vi "Start_10_July.vi"() -> ()   [LabVIEW 2015]
uses:
  gfitsio/gfitsio-refnum.ctl
  SystemUtil/Command.ctl
  Instance          11 21Saved   Start_10_July .vi
  Instance          12 21Saved   Start_10_July .vi
panel:
  in  "Zoom Window Width (1/x)":u32=10
  out "max index(es)":i32
  out "max index(es) 2":i32
  in  "Resolution Factor":u16=4
  out "Spectrum Status":string
  out "Image Buffer Info.":T1
  out "error IO":errorcluster
  out "Raw Spectrum Array":dbl[](array[numeric])
  in  "# of rows at a time":dbl=1.0
  in  "Black Square":picture
  in  "Image Buffer":i32[][](array[numeric])
  out "Column Cut Cursor Position":dbl
  out "Raw Image Buffer 1":i16[][](array[numeric])
  out "Raw Data":T2
  out "gfits refnum":T3
  in  "Tab Control":T4(tab)
  in  "Autoscale":bool
  in  "Image Display Resolution":u16(ring)=2 items=["High", "Medium", "Low"]
  in  "Send Object Offset Position":bool
  in  "Send Target Offset Position":bool
  in  "Automatic Acquisition?":bool=TRUE caption="Display:"
  in  "Display Directions?":bool caption="Display:"
  in  "Redraw":bool
  in  "Zoom Out":bool
  in  "Zoom In":bool
  out "Y":dbl format="%5.1f"
  out "X":dbl format="%5.1f"
  out "Value":dbl
  out "Zoom Window":i16[][](graph) caption="0051.NGC2808_300line.fits"
  out "Compass":picture
  out "Image Status":string
  in  "Image Scale Stretch":cluster{dbl, dbl}(slide)={0.0, 1.4018691588785046} scale=0.0..100.0
  in  "Image":dbl[][](graph)=[[10.0, 5.0, 0.0], [0.0, 6.0, 7.0]] caption="Image Buffer"
  out "Calib Spec":cluster{dbl, dbl}[](graph) caption="Spectrum Centered at Row 53"
  in  "Show x scale in:":i32(listbox)
  in  "Refresh Spectrum":bool
  in  "Aperture Width (pix)":dbl=5.0
  out "Cut Along Column":i16[](graph)
  in  "Cut Along Column #":dbl min=0.0 max=2071.0
  in  "Refresh Spatial Cut":bool
  out "Minimum Pix Value":dbl
  out "Maximum Pix Value":dbl
  out "Avg Pix Value":dbl format="%#.1f"
  in  "Header Scroll":dbl(slide)=100.0 scale=0.0..100.0
  out "FITS Header":string[](array[string])
  in  "CommandQ":string="QUICKLOOK_Q"
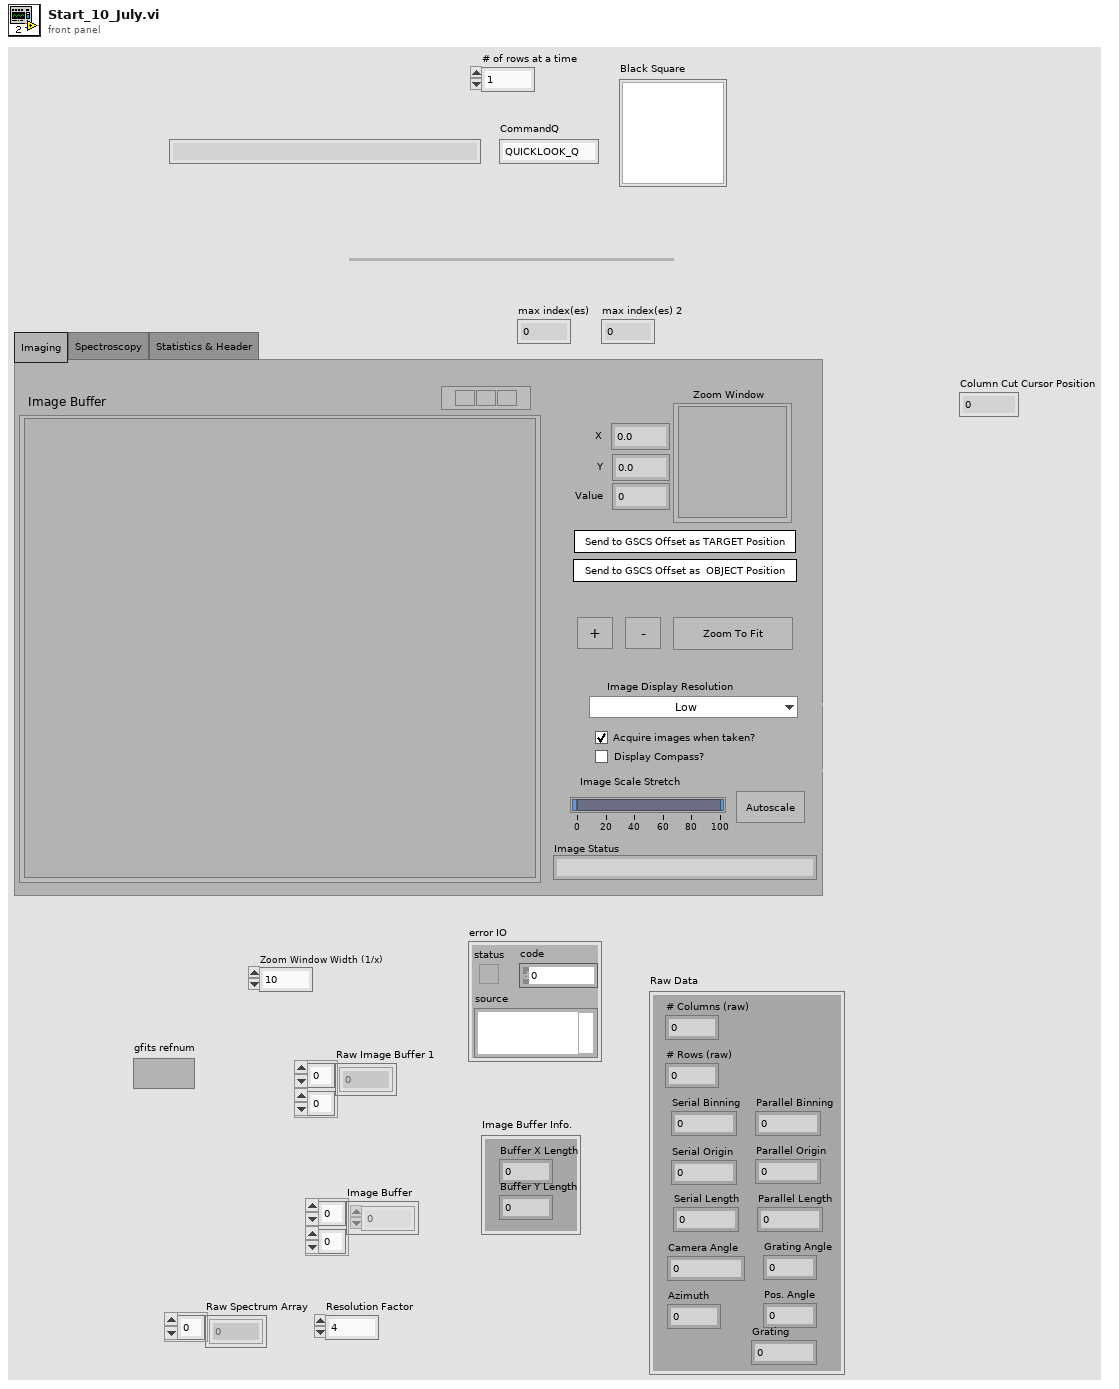
[diagram p1: front panel]
types:
  T1 = cluster{"Buffer X Length":dbl, "Buffer Y Length ":dbl}
  T2 = cluster{"# Columns (raw) ":dbl, "# Rows (raw)":dbl, "Serial Origin":dbl, "Parallel Origin":dbl, "Camera Angle":dbl, "Grating Angle":dbl, "Serial Binning":dbl, "Parallel Binning":dbl, "Azimuth":dbl, "Serial Length":dbl, "Parallel Length":dbl, "Pos. Angle":dbl, "Grating":dbl}
  T3 = typedef "gfitsio-refnum.ctl" = refnum<k1>
  T4 = enum32{"Imaging", "Spectroscopy", "Statistics & Header"}
  T5 = typedef "Command.ctl" = cluster{"Command":string, "Parameter":string}
  T6 = enum16{"open", "open or create", "create or replace", "create", "open (read only)"}
  T7 = cluster{"Width":u16, "Style":enum32{"Solid", "Dash", "Dot", "DashDot", "DashDotDot"}}
  T8 = enum32{"existing file", "new file", "new or existing file", "existing dir", "new dir", "new or existing dir", "existing file (use LLBs)", "new file (use LLBs)", "new or existing file (use LLBs)", "new or existing file or directory (use LLBs)"}
  T9 = typedef "LVRangeTypeDef.ctl" = cluster{"Minimum":dbl, "Maximum":dbl, "Increment":dbl, "Minor Increment":dbl, "Start":dbl}
  T10 = typedef "LVPoint32TypeDef.ctl" = cluster{"Horizontal":i32, "Vertical":i32}
  T11 = typedef "LVPointDoubleTypeDef.ctl" = cluster{"Cursor X":dbl, "Cursor Y":dbl}
  T12 = cluster{"Font Name:":string, "Size":i16, "Strikeout?":bool, "Italic?":bool, "Underline?":bool, "Outline?":bool, "Shadow?":bool, "Bold?":bool}
  T13 = cluster{"horizontal":enum16{"left", "center", "right"}, "vertical":enum16{"top", "center", "bottom"}}
  T14 = enum16{"User-specified Font", "Application Font", "System Font", "Dialog Font"}
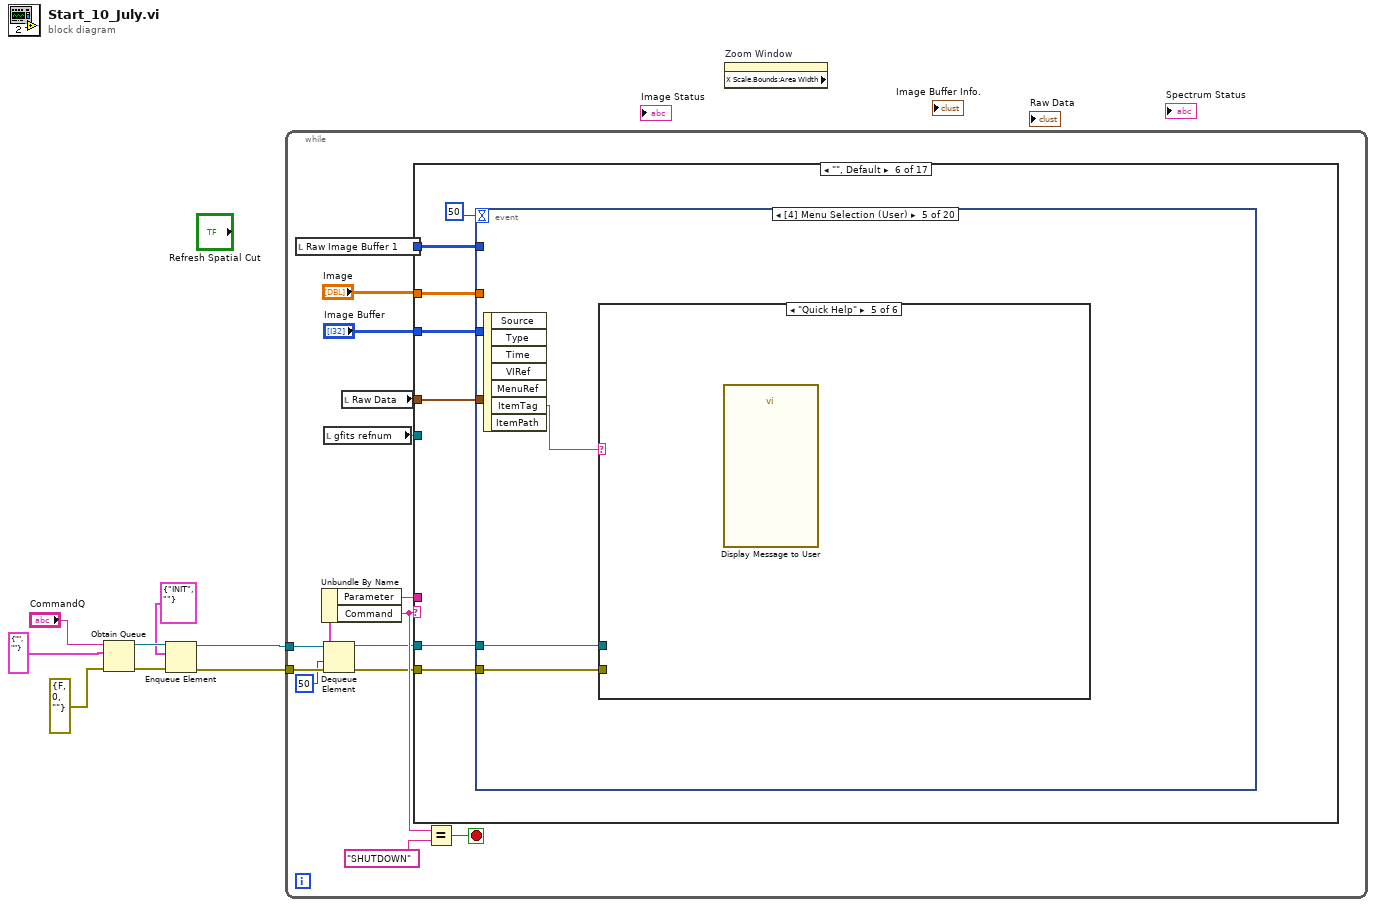
[diagram p0: block diagram]
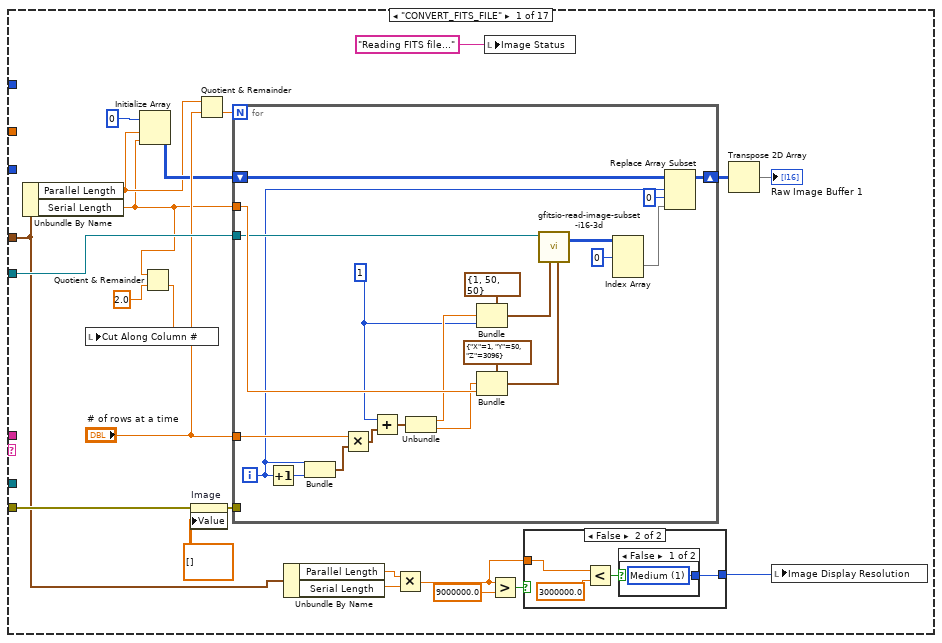
[diagram p2: hidden frame]
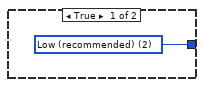
[diagram p3: hidden frame]
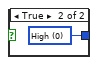
[diagram p4: hidden frame]
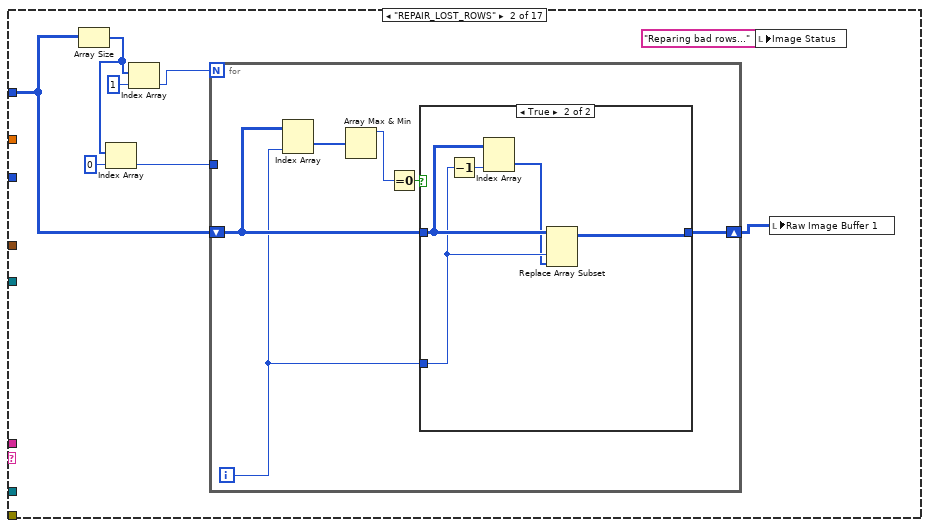
[diagram p5: hidden frame]
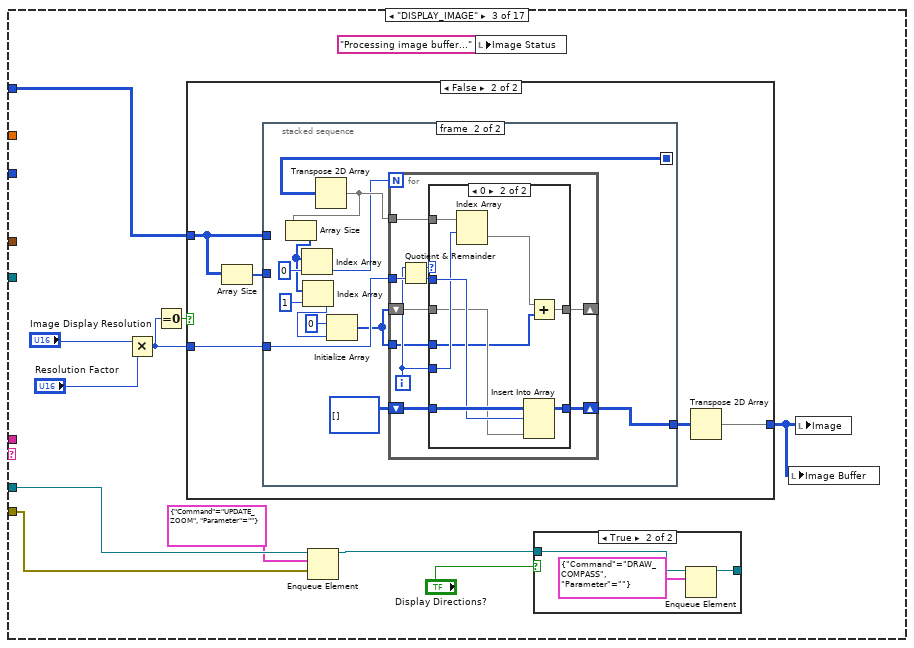
[diagram p7: hidden frame]
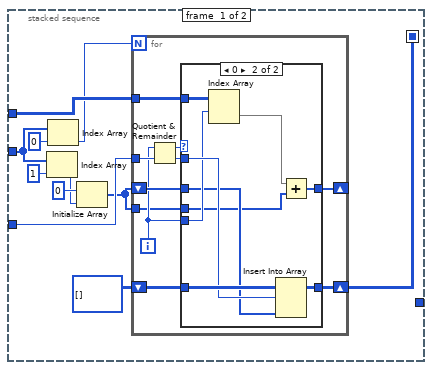
[diagram p10: hidden frame]
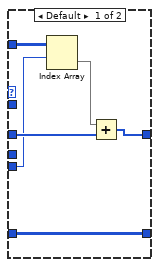
[diagram p11: hidden frame]
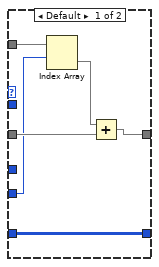
[diagram p12: hidden frame]
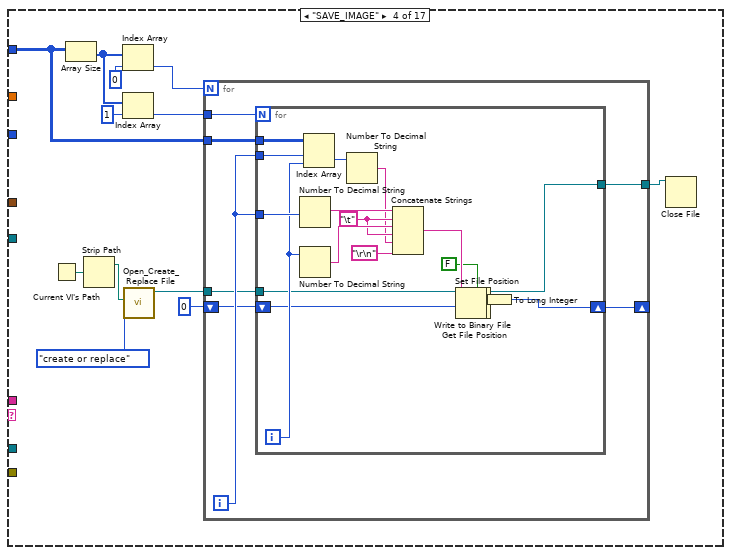
[diagram p13: hidden frame]
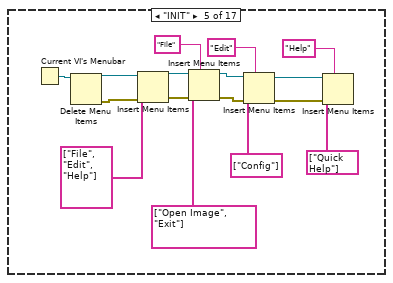
[diagram p14: hidden frame]
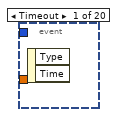
[diagram p15: hidden frame]
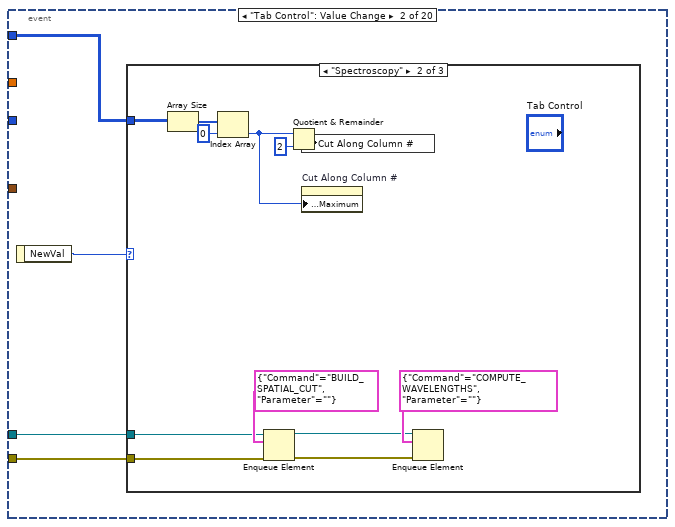
[diagram p16: hidden frame]
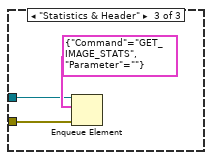
[diagram p18: hidden frame]
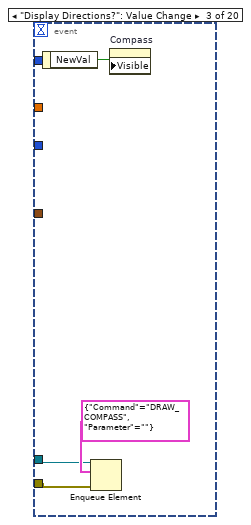
[diagram p19: hidden frame]
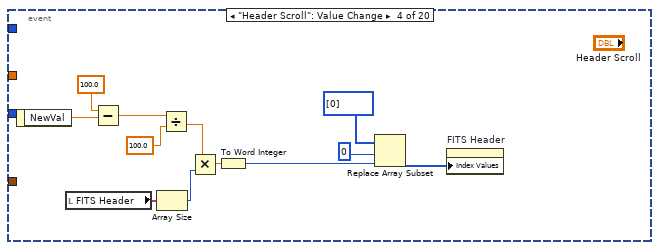
[diagram p20: hidden frame]
diagram:
  n1 = Obtain Queue(name (unnamed)="CommandQ", element data type=T5 {"Command"="", "Parameter"=""} ("Command"), error in (no error)=errorcluster {"status"=FALSE, "code"=0, "source"=""}) -> (queue out=w6:refnum<queue>, error out=w5:errorcluster)  [unwired: 2 in, 1 out]
  n2 = Enqueue Element(queue=w6, element=T5 {"Command"="INIT", "Parameter"=""}, error in (no error)=w5) -> (queue out=w3:refnum<queue>, error out=w2:errorcluster)  [unwired: 1 in, 1 out]
  n3 = while {
    tunnel: w2 -> [w23]
    tunnel: w3 -> [w22]
    stop <- w19 stop-if-true
    n4 = local read "Raw Image Buffer 1"() -> (w9:i16[][])
    n5 = local read "gfits refnum"() -> (w13:T3)
    n6 = Dequeue Element(queue=w22, timeout in ms (-1)=50, error in (no error)=w23) -> (queue out=w16:refnum<queue>, element=w21:T5, error out=w17:errorcluster)  [unwired: 1 out]
    n7 = Unbundle By Name(w21) -> ("Parameter"=w14:string, "Command"=w18:string)
    n8 = local read "Raw Data"() -> (w12:T2)
    n9 = case shown="\"\", Default" w18 {
      tunnel: w17 -> [w36 _ w94 _ _ w249 w652 _ _ _ _ _ _ _ w990 w1020 _]
      tunnel: w16 -> [_ _ w97 _ _ w250 w653 _ _ _ _ _ _ _ w989 _ _]
      tunnel: w14 -> [_ _ _ _ _ _ _ _ _ _ _ _ _ _ w988 _ _]
      tunnel: "Image" -> [_ _ _ _ _ w248 _ _ _ _ _ _ _ _ _ _ _]
      tunnel: w13 -> [w45 _ _ _ _ _ _ _ _ _ _ _ _ _ _ w1021 _]
      tunnel: w12 -> [w30 _ _ _ _ w247 w651 _ _ _ w841 w909 _ w971 _ w1018 _]
      tunnel: "Image Buffer" -> [_ _ _ _ _ w246 _ _ _ _ _ _ _ _ _ _ _]
      tunnel: w9 -> [_ w78 w101 w198 _ w245 _ _ w777 w783 _ _ w964 w967 _ _ w1091]
      frame "CONVERT_FITS_FILE" {
        n10 = Unbundle By Name(w30) -> ("Parallel Length"=w32:dbl, "Serial Length"=w31:dbl)
        n11 = Initialize Array(i16 0 ("element"), w32, w31) -> (w34:i16[][])
        n12 = Quotient & Remainder(x=w31, y=2.0) -> (floor(x/y)=w39:dbl)  [unwired: 1 out]
        n13 = local write "Cut Along Column #"(w39) -> ()
        n14 = property on="Image" class="IntGraph (strict)"(error in=w36, "Value"=dbl[][] [] ("Image")) -> (error out=w37:errorcluster)  [unwired: 1 in, 1 out]
        n15 = Quotient & Remainder(x=w32, y="# of rows at a time") -> (floor(x/y)=w44:dbl)  [unwired: 1 out]
        n16 = for {
          N: w44 -> [_]
          tunnel: w31 -> [w72]
          tunnel: w45 -> [w61]
          tunnel: "# of rows at a time" -> [w71]
          shift-right: [w57] -> w41
          shift-left: w34 -> [w56]
          tunnel: w37 -> [_]
          i -> [w55]
          w64 = 1
          n17 = Increment(x=w55) -> (x+1=w68:i32)
          n18 = Bundle(w55, w68) -> (w69:cluster{i32, i32})  [unwired: 1 in]
          n19 = Multiply(x=w71, y=w69) -> (x*y=w70:cluster{dbl, dbl})
          n20 = Add(x=w64, y=w70) -> (x+y=w67:cluster{dbl, dbl})
          n21 = Unbundle(w67) -> (w65:dbl, w66:dbl)
          n22 = Bundle(cluster=cluster{"X":i32, "Y":i32, "Z":i32} {"X"=1, "Y"=50, "Z"=50} ("fpixel (1,1,1)"), "Y"=w65, "Z"=w64) -> (w60:cluster{"X":i32, "Y":i32, "Z":i32})  [unwired: 1 in]
          n23 = Bundle(cluster=cluster{"X":i32, "Y":i32, "Z":i32} {"X"=1, "Y"=50, "Z"=3096} ("lpixel (-1,-1,-1: rest)"), "Y"=w66, "Z"=w72) -> (w59:cluster{"X":i32, "Y":i32, "Z":i32})  [unwired: 1 in]
          n24 = call "gfitsio-read-image-subset-i16-3d.vi"("lpixel (-1,-1,-1: rest)"=w59, "fpixel (1,1,1)"=w60, "gfits refnum"=w61) -> ("data"=w58:i16[][][])  [unwired: 5 in, 3 out]
          n25 = Index Array(array=w58, index (dim 0)=i16 0 ("index (page)")) -> (element=w54:i16[][])  [unwired: 2 in]
          n26 = Replace Array Subset(array=w56, new element=w54, index (row)=w55, index (col)=0 ("disabled index (col)")) -> (w57:i16[][])
        }
        n27 = Unbundle By Name(w30) -> ("Parallel Length"=w29:dbl, "Serial Length"=w28:dbl)
        n28 = Multiply(x=w29, y=w28) -> (x*y=w24:dbl)
        n29 = local write "Image Status"("Reading FITS file..." ("Status")) -> ()
        n30 = Greater?(x=w24, y=9000000.0) -> (0:w26:bool)
        n31 = case shown="False" w26 {
          tunnel: [w46 w47] -> w25
          tunnel: w24 -> [_ w49]
          frame True {
            w46 = u16 2 items=["High", "Medium", "Low (recommended)"] ("Image Display Resolution")
          }
          frame False {
            n32 = Less?(x=w49, y=3000000.0) -> (x < y?=w50:bool)
            n33 = case shown="False" w50 {
              tunnel: [w51 w52] -> w47
              frame False {
                w51 = u16 1 items=["High", "Medium", "Low (recommended)"] ("Image Display Resolution")
              }
              frame True {
                w52 = u16 0 items=["High", "Medium", "Low (recommended)"] ("Image Display Resolution")
              }
            }
          }
        }
        n34 = Transpose 2D Array(2D array=w41) -> (transposed array=→"Raw Image Buffer 1":i16[][])
        n35 = local write "Image Display Resolution"(w25) -> ()
      }
      frame "REPAIR_LOST_ROWS" {
        n36 = Array Size(array=w78) -> (size(s)=w75:i32[])
        n37 = Index Array(array=w75, index=0) -> (element=w74:i32)
        n38 = Index Array(array=w75, index=1) -> (element=w79:i32)
        n39 = for {
          N: w79 -> [_]
          shift-right: [w87] -> w80
          shift-left: w78 -> [w86]
          tunnel: w74 -> [_]
          i -> [w85]
          n40 = Index Array(array=w86, index (col)=w85) -> (element=w84:i16[])  [unwired: 1 in]
          n41 = Array Max & Min(array=w84) -> (max value=w82:i16)  [unwired: 3 out]
          n42 = Equal To 0?(x=w82) -> (x = 0?=w83:bool)
          n43 = case shown="True" w83 {
            tunnel: w85 -> [_ w90]
            tunnel: w86 -> [w88 w92]
            tunnel: [w88 w93] -> w87
            frame False {
            }
            frame True {
              n44 = Decrement(x=w90) -> (x-1=w91:i32)
              n45 = Index Array(array=w92, index (col)=w91) -> (element=w89:i16[])  [unwired: 1 in]
              n46 = Replace Array Subset(array=w92, new element=w89, index (col)=w90) -> (w93:i16[][])  [unwired: 1 in]
            }
          }
        }
        n47 = local write "Image Status"("Reparing bad rows..." ("Image Status")) -> ()
        n48 = local write "Raw Image Buffer 1"(w80) -> ()
      }
      frame "DISPLAY_IMAGE" {
        n49 = Multiply(x="Image Display Resolution", y="Resolution Factor") -> (x*y=w102:u16)
        n50 = Equal To 0?(x=w102) -> (x = 0?=w103:bool)
        n51 = case shown="False" w103 {
          tunnel: w101 -> [w110 w114]
          tunnel: w102 -> [_ w112]
          tunnel: [w110 w111] -> w99
          frame True {
          }
          frame False {
            n52 = Array Size(array=w114) -> (size(s)=w115:i32[])
            n53 = stacked-sequence {
              seq-local: [w124 _] -> [_ w161]
              tunnel: w114 -> [w126 _]
              tunnel: w115 -> [w118 _]
              tunnel: w112 -> [w122 w158]
              tunnel: [_ w162] -> w113
              frame #0 {
                n54 = Index Array(array=w118, index=1) -> (element=w117:i32)
                n55 = Index Array(array=w118, index=0) -> (element=w120:i32)
                n56 = Initialize Array(0 ("element"), w117) -> (w116:i32[])
                n57 = for {
                  N: w120 -> [_]
                  tunnel: w126 -> [w136]
                  shift-right: [w134] -> w124
                  shift-left: i32[][] [] -> [w135]
                  tunnel: w122 -> [w133]
                  shift-right: [w129] -> _
                  shift-left: w116 -> [w130]
                  tunnel: w116 -> [w127]
                  i -> [w128]
                  n58 = Quotient & Remainder(x=w128, y=w133) -> (x-y*floor(x/y)=w132:i32, floor(x/y)=w131:i32)
                  n59 = case shown="0" w132 {
                    tunnel: w136 -> [w142 w151]
                    tunnel: w128 -> [w138 w147]
                    tunnel: w135 -> [w137 w150]
                    tunnel: [w137 w149] -> w134
                    tunnel: w131 -> [_ w148]
                    tunnel: w130 -> [w140 w146]
                    tunnel: [w139 w144] -> w129
                    tunnel: w127 -> [_ w143]
                    frame Default {
                      n60 = Index Array(array=w142, index (row)=w138) -> (element=w141:i16[])  [unwired: 1 in]
                      n61 = Add(x=w141, y=w140) -> (x+y=w139:i32[])
                    }
                    frame 0 {
                      n62 = Index Array(array=w151, index (row)=w147) -> (element=w145:i16[])  [unwired: 1 in]
                      n63 = Insert Into Array(array=w150, index (row)=w148, new element=w146) -> (w149:i32[][])  [unwired: 1 in]
                      n64 = Add(x=w145, y=w143) -> (x+y=w144:i32[])
                    }
                  }
                }
              }
              frame #1 {
                n65 = Transpose 2D Array(2D array=w161) -> (transposed array=w159:i32[][])
                n66 = Array Size(array=w159) -> (size(s)=w153:i32[])
                n67 = Index Array(array=w153, index=0) -> (element=w156:i32)
                n68 = Index Array(array=w153, index=1) -> (element=w154:i32)
                n69 = Initialize Array(0 ("element"), w154) -> (w152:i32[])
                n70 = for {
                  N: w156 -> [_]
                  tunnel: w159 -> [w173]
                  shift-right: [w166] -> w162
                  shift-left: i32[][] [] -> [w167]
                  shift-right: [w172] -> _
                  shift-left: w152 -> [w171]
                  tunnel: w158 -> [w168]
                  tunnel: w152 -> [w164]
                  i -> [w165]
                  n71 = Quotient & Remainder(x=w165, y=w168) -> (x-y*floor(x/y)=w170:i32, floor(x/y)=w169:i32)
                  n72 = case shown="0" w170 {
                    tunnel: w173 -> [w179 w188]
                    tunnel: w165 -> [w175 w184]
                    tunnel: w167 -> [w174 w187]
                    tunnel: [w174 w186] -> w166
                    tunnel: w169 -> [_ w185]
                    tunnel: w171 -> [w177 w183]
                    tunnel: [w176 w181] -> w172
                    tunnel: w164 -> [_ w180]
                    frame Default {
                      n73 = Index Array(array=w179, index (row)=w175) -> (element=w178:i32[])  [unwired: 1 in]
                      n74 = Add(x=w178, y=w177) -> (x+y=w176:i32[])
                    }
                    frame 0 {
                      n75 = Index Array(array=w188, index (row)=w184) -> (element=w182:i32[])  [unwired: 1 in]
                      n76 = Insert Into Array(array=w187, index (row)=w185, new element=w183) -> (w186:i32[][])  [unwired: 1 in]
                      n77 = Add(x=w182, y=w180) -> (x+y=w181:i32[])
                    }
                  }
                }
              }
            }
            n78 = Transpose 2D Array(2D array=w113) -> (transposed array=w111:i32[][])
          }
        }
        n79 = Enqueue Element(queue=w97, element=T5 {"Command"="UPDATE_ZOOM", "Parameter"=""}, error in (no error)=w94) -> (queue out=w96:refnum<queue>)  [unwired: 1 in, 2 out]
        n80 = local write "Image Status"("Processing image buffer..." ("Status")) -> ()
        n81 = case shown="True" "Display Directions?" {
          tunnel: w96 -> [w106 w108]
          tunnel: [w106 w107] -> _
          frame False {
          }
          frame True {
            n82 = Enqueue Element(queue=w108, element=T5 {"Command"="DRAW_COMPASS", "Parameter"=""}) -> (queue out=w107:refnum<queue>)  [unwired: 2 in, 2 out]
          }
        }
        n83 = local write "Image Buffer"(w99) -> ()
        n84 = local write "Image"(w99) -> ()
      }
      frame "SAVE_IMAGE" {
        n85 = Current VI's Path() -> (path=w193:path)
        n86 = Array Size(array=w198) -> (size(s)=w196:i32[])
        n87 = Strip Path(path=w193) -> (stripped path=w192:path)  [unwired: 1 out]
        n88 = Index Array(array=w196, index=0) -> (element=w199:i32)
        n89 = Index Array(array=w196, index=1) -> (element=w195:i32)
        n90 = call <vilib>:"Open_Create_Replace File.vi"("function (open:0)"=T6."create or replace", "start path  (Not A Path)"=w192) -> ("refnum"=w191:refnum<file>)  [unwired: 6 in, 3 out]
        n91 = for {
          N: w199 -> [_]
          tunnel: w198 -> [w207]
          tunnel: w195 -> [w206]
          tunnel: w191 -> [w204]
          tunnel: [w203] -> w190
          shift-right: [w201] -> _
          shift-left: 0 ("pos offset (0)") -> [w202]
          i -> [w205]
          n92 = for {
            N: w206 -> [_]
            tunnel: w207 -> [w228]
            tunnel: w205 -> [w227]
            tunnel: w205 -> [w226]
            tunnel: w204 -> [w218]
            tunnel: [w217] -> w203
            shift-right: [w215] -> w201
            shift-left: w202 -> [w216]
            i -> [w221]
            w223 = "\t"
            n93 = Number To Decimal String(number=w226) -> (decimal integer string=w225:string)  [unwired: 1 in]
            n94 = Number To Decimal String(number=w221) -> (decimal integer string=w224:string)  [unwired: 1 in]
            n95 = Index Array(array=w228, index (row)=w227, index (col)=w221) -> (element=w222:i16)
            n96 = Number To Decimal String(number=w222) -> (decimal integer string=w220:string)  [unwired: 1 in]
            n97 = Concatenate Strings(w225, w223, w224, w223, w220, "\r\n") -> (w219:string)
            n98 = Set File Position(offset (in bytes) (0)=w216, refnum=w218) -> (refnum out=w213:refnum<file>, error out=w212:errorcluster)  [unwired: 2 in]
            n99 = Write to Binary File(file (use dialog)=w213, data=w219, error in=w212, 5:FALSE ("prepend array or string size? (T)")) -> (refnum out=w211:refnum<file>, error out=w210:errorcluster)  [unwired: 2 in, 1 out]
            n100 = Get File Position(4:w210, 7:w211) -> (2:w209:i64, 3:w217:refnum<file>)  [unwired: 1 out]
            n101 = To Long Integer(number=w209) -> (32bit integer=w215:i32)
          }
        }
        n102 = Close File(refnum=w190) -> ()  [unwired: 1 in, 2 out]
      }
      frame "INIT" {
        n103 = Current VI's Menubar() -> (w244:refnum<k9>)
        n104 = Delete Menu Items(9:w244) -> (0:w242:errorcluster, 3:w243:refnum<k9>)  [unwired: 3 in]
        n105 = Insert Menu Items(6:w242, 8:string[] ["File", "Edit", "Help"] ("item names"), 9:w243) -> (0:w237:errorcluster, 3:w240:refnum<k9>)  [unwired: 3 in, 1 out]
        n106 = Insert Menu Items(5:"File" ("menu tag"), 6:w237, 8:string[] ["Open Image", "Exit"] ("item names"), 9:w240) -> (0:w235:errorcluster, 3:w236:refnum<k9>)  [unwired: 2 in, 1 out]
        n107 = Insert Menu Items(5:"Edit" ("menu tag"), 6:w235, 8:string[] ["Config"] ("item names"), 9:w236) -> (0:w231:errorcluster, 3:w232:refnum<k9>)  [unwired: 2 in, 1 out]
        n108 = Insert Menu Items(5:"Help" ("menu tag"), 6:w231, 8:string[] ["Quick Help"] ("item names"), 9:w232) -> ()  [unwired: 2 in, 3 out]
      }
      frame "", Default {
        n109 = event shown="[4] Menu Selection (User)" {
          selector: _ -> [_ _ _ _ _ _ _ _ _ _ _ _ _ _ _ _ _ _ _ _]
          dyn-events: _ -> [_ _ _ _ _ _ _ _ _ _ _ _ _ _ _ _ _ _ _ _]
          timeout: 50 -> [_ _ _ _ _ _ _ _ _ _ _ _ _ _ _ _ _ _ _ _]
          tunnel: w250 -> [_ w253 w271 _ w288 _ w317 w320 w324 _ _ _ _ w587 w596 w613 w615 w618 _ w648]
          tunnel: w249 -> [_ w254 w272 _ w287 _ w318 w321 w325 _ _ _ _ w588 w598 w612 w616 w619 _ w647]
          tunnel: w248 -> [_ _ _ _ _ _ _ _ w326 _ _ _ _ _ _ _ _ w620 _ _]
          tunnel: w247 -> [_ _ _ _ _ _ _ _ w323 _ _ _ _ _ _ _ _ _ _ _]
          tunnel: w246 -> [_ _ _ _ _ _ _ _ _ _ _ _ _ _ _ _ _ _ _ _]
          tunnel: w245 -> [_ w252 _ _ _ _ _ _ _ _ _ _ _ _ _ _ _ _ _ _]
          event Timeout {
            n110 = event-data() -> ()  [unwired: 1 in, 2 out]
          }
          event "Tab Control": Value Change {
            n111 = event-data() -> ("NewVal"=w255:T4)  [unwired: 1 in]
            n112 = case shown="\"Spectroscopy\"" w255 {
              tunnel: w252 -> [_ w267 _]
              tunnel: w254 -> [_ w260 w269]
              tunnel: w253 -> [_ w259 w268]
              frame "Imaging", Default {
              }
              frame "Spectroscopy" {
                n113 = Array Size(array=w267) -> (size(s)=w266:i32[])
                n114 = Index Array(array=w266, index=0) -> (element=w262:i32)
                n115 = Enqueue Element(queue=w259, element=T5 {"Command"="BUILD_SPATIAL_CUT", "Parameter"=""}, error in (no error)=w260) -> (queue out=w256:refnum<queue>, error out=w257:errorcluster)  [unwired: 1 in, 1 out]
                n116 = Quotient & Remainder(x=w262, y=2) -> (floor(x/y)=w263:i32)  [unwired: 1 out]
                n117 = local write "Cut Along Column #"(w263) -> ()
                n118 = property on="Cut Along Column #" class="DigNum (strict)"("Data Entry Limits:Maximum"=w262) -> ()  [unwired: 2 in, 2 out]
                n119 = Enqueue Element(queue=w256, element=T5 {"Command"="COMPUTE_WAVELENGTHS", "Parameter"=""}, error in (no error)=w257) -> ()  [unwired: 1 in, 3 out]
              }
              frame "Statistics & Header" {
                n120 = Enqueue Element(queue=w268, element=T5 {"Command"="GET_IMAGE_STATS", "Parameter"=""}, error in (no error)=w269) -> ()  [unwired: 1 in, 3 out]
              }
            }
          }
          event "Display Directions?": Value Change {
            n121 = event-data() -> ("NewVal"=w274:bool)  [unwired: 1 in]
            n122 = Enqueue Element(queue=w271, element=T5 {"Command"="DRAW_COMPASS", "Parameter"=""}, error in (no error)=w272) -> ()  [unwired: 1 in, 3 out]
            n123 = property on="Compass" class="Pict"("Visible"=w274) -> ()  [unwired: 2 in, 2 out]
          }
          event "Header Scroll": Value Change {
            n124 = event-data() -> ("NewVal"=w284:dbl)  [unwired: 1 in]
            n125 = local read "FITS Header"() -> (w286:string[])
            n126 = Subtract(x=100.0, y=w284) -> (x-y=w276:dbl)
            n127 = Array Size(array=w286) -> (size(s)=w283:i32)
            n128 = Divide(x=w276, y=100.0) -> (x/y=w275:dbl)
            n129 = Multiply(x=w275, y=w283) -> (x*y=w279:dbl)
            n130 = To Word Integer(number=w279) -> (16bit integer=w278:i16)
            n131 = Replace Array Subset(array=u32[] [0] ("Index Values"), new element=w278, index=0) -> (w280:u32[])
            n132 = property on="FITS Header" class="Arr (strict)"("Index Values"=w280) -> ()  [unwired: 2 in, 2 out]
          }
          event Menu Selection (User) {
            n133 = event-data() -> ("ItemTag"=w289:string)  [unwired: 1 in, 6 out]
            n134 = case shown="\"Quick Help\"" w289 {
              tunnel: w288 -> [_ w292 w300 _ _ w313]
              tunnel: w287 -> [_ w291 w301 _ _ w312]
              frame "", Default {
              }
              frame "Exit" {
                n135 = Enqueue Element(queue=w292, element=T5 {"Command"="SHUTDOWN", "Parameter"=""}, error in (no error)=w291) -> ()  [unwired: 1 in, 3 out]
              }
              frame "Open Image" {
                (unwired) T8."existing file" ("select mode (2)")
                n136 = File Dialog(5:"Open Image" ("button label"), 6:"*.fits" ("default name"), 7:"Open Image" ("prompt")) -> (0:w293:errorcluster, 1:w297:bool, 3:w298:path)  [unwired: 4 in, 1 out]
                n137 = Unbundle(w293) -> ()  [unwired: 3 out]
                n138 = Path To String(path=w298) -> (string=w299:string)
                n139 = case shown="False" w297 {
                  tunnel: w301 -> [_ w307]
                  tunnel: w300 -> [_ w306]
                  tunnel: w299 -> [_ w304]
                  frame True {
                  }
                  frame False {
                    n140 = Bundle By Name(cluster=T5 {"Command"="", "Parameter"=""} ("element"), "Command"="OPEN_FITS_FILE", "Parameter"=w304) -> (w305:T5)
                    n141 = Enqueue Element(queue=w306, element=w305, error in (no error)=w307) -> ()  [unwired: 1 in, 3 out]
                  }
                }
              }
              frame "Config" {
                n142 = call "Configuration Parameters"() -> ("Rows to read in at a time"=w310:dbl)  [unwired: 15 in, 4 out]
                n143 = Equal To 0?(x=w310) -> (x = 0?=w311:bool)
                n144 = Select(t=5.0, s=w311, f=w310) -> (s? t:f=w308:dbl)
                n145 = local write "# of rows at a time"(w308) -> ()
              }
              frame "Quick Help" {
                n146 = call "Display Message to User"() -> ()  [unwired: 10 in, 2 out]
              }
              frame "Save" {
                n147 = Enqueue Element(queue=w313, element=T5 {"Command"="SAVE_IMAGE", "Parameter"=""}, error in (no error)=w312) -> ()  [unwired: 1 in, 3 out]
              }
            }
          }
          event "Autoscale": Value Change {
            n148 = event-data() -> ()  [unwired: 1 in, 6 out]
            n149 = property on="Image" class="IntGraph (strict)"("Z Scale.Scale Fit"=u8 1) -> ()  [unwired: 2 in, 2 out]
            n150 = local write "Autoscale"(FALSE ("Autoscale")) -> ()
          }
          event "Image Display Resolution": Value Change {
            n151 = event-data() -> ()  [unwired: 1 in, 6 out]
            n152 = Enqueue Element(queue=w317, element=T5 {"Command"="DISPLAY_IMAGE", "Parameter"=""}, error in (no error)=w318) -> ()  [unwired: 1 in, 3 out]
          }
          event "Redraw": Mouse Down {
            n153 = event-data() -> ()  [unwired: 1 in, 8 out]
            n154 = Enqueue Element(queue=w320, element=T5 {"Command"="DISPLAY_IMAGE", "Parameter"=""}, error in (no error)=w321) -> ()  [unwired: 1 in, 3 out]
          }
          event Key Down {
            n155 = event-data() -> ("Char"=w327:i16)  [unwired: 1 in]
            n156 = case shown="116" w327 {
              selector: w327 -> [_ _ w342 _ _ _ _ _]
              tunnel: w326 -> [_ _ _ _ _ _ _ _]
              tunnel: w325 -> [_ _ w338 w361 w430 _ w490 _]
              tunnel: w324 -> [_ _ w337 w362 w431 _ w489 _]
              tunnel: w323 -> [_ _ _ _ _ _ _ _]
              frame 0 {
              }
              frame Default {
              }
              frame 105..108 {
                w332 = u16 1 ("t")
                n157 = local read "Image Display Resolution"() -> (w335:u16)
                n158 = local read "Resolution Factor"() -> (w328:u16)
                n159 = property on="Image" class="IntGraph (strict)"() -> ("Cursor.Cursor Position:Cursor X"=w330:dbl)  [unwired: 2 in, 2 out]
                n160 = property on="Image" class="IntGraph (strict)"() -> ("Cursor.Cursor Position:Cursor Y"=w329:dbl)  [unwired: 2 in, 2 out]
                n161 = Enqueue Element(queue=w337, element=T5 {"Command"="UPDATE_ZOOM", "Parameter"=""}, error in (no error)=w338) -> ()  [unwired: 1 in, 3 out]
                n162 = Multiply(x=w335, y=w328) -> (x*y=w336:u16)
                n163 = Equal To 0?(x=w335) -> (x = 0?=w334:bool)
                n164 = Select(t=w332, s=w334, f=w336) -> (s? t:f=w333:u16)
                n165 = Divide(x=w332, y=w333) -> (x/y=w331:dbl)
                n166 = case shown="105" w342 {
                  tunnel: w330 -> [w344 w347 w352 w355 w360]
                  tunnel: [w344 w346 w352 w354 w360] -> w341
                  tunnel: w329 -> [w343 w348 w350 w356 w358]
                  tunnel: [w343 w348 w349 w356 w357] -> w340
                  tunnel: w331 -> [_ w345 w351 w353 w359]
                  frame 0, Default {
                  }
                  frame 108 {
                    n167 = Add(x=w347, y=w345) -> (x+y=w346:dbl)
                  }
                  frame 105 {
                    n168 = Add(x=w350, y=w351) -> (x+y=w349:dbl)
                  }
                  frame 106 {
                    n169 = Subtract(x=w355, y=w353) -> (x-y=w354:dbl)
                  }
                  frame 107 {
                    n170 = Subtract(x=w358, y=w359) -> (x-y=w357:dbl)
                  }
                }
                n171 = property on="Image" class="IntGraph (strict)"("Cursor.Cursor Position:Cursor X"=w341) -> ()  [unwired: 2 in, 2 out]
                n172 = property on="Image" class="IntGraph (strict)"("Cursor.Cursor Position:Cursor Y"=w340) -> ()  [unwired: 2 in, 2 out]
              }
              frame 114 {
                n173 = local read "Zoom Window"() -> (w368:i16[][])
                n174 = Array Size(array=w368) -> (size(s)=w364:i32[])
                n175 = Index Array(array=w364, index=1) -> (element=w363:i32)
                n176 = Index Array(array=w364, index=0) -> (element=w366:i32)
                n177 = stacked-sequence {
                  seq-local: [w369 _ _ _] -> [_ _ w407 _]
                  seq-local: [_ w382 _ _] -> [_ _ w408 _]
                  seq-local: [_ _ w395 _] -> [_ _ _ w422]
                  tunnel: w368 -> [w375 w386 _ _]
                  tunnel: w366 -> [w372 w385 _ _]
                  tunnel: w363 -> [w371 w384 _ _]
                  tunnel: w362 -> [_ _ _ w418]
                  tunnel: w361 -> [_ _ _ w417]
                  frame #0 {
                    n178 = Initialize Array(0 ("element"), w371) -> (w374:i32[])
                    n179 = for {
                      N: w372 -> [_]
                      tunnel: w375 -> [w381]
                      shift-right: [w380] -> w370
                      shift-left: w374 -> [w378]
                      i -> [w376]
                      n180 = Index Array(array=w381, index (row)=w376) -> (element=w379:i16[])  [unwired: 1 in]
                      n181 = Add(x=w379, y=w378) -> (x+y=w377:i32[])
                      n182 = Replace Array Subset(array=w378, new element=w377) -> (w380:i32[])  [unwired: 1 in]
                    }
                    n183 = Array Max & Min(array=w370) -> (max index (indices)=w369:i32)  [unwired: 3 out]
                  }
                  frame #1 {
                    n184 = Initialize Array(0 ("element"), w385) -> (w388:i32[])
                    n185 = for {
                      N: w384 -> [_]
                      tunnel: w386 -> [w394]
                      shift-right: [w393] -> w383
                      shift-left: w388 -> [w390]
                      i -> [w389]
                      n186 = Index Array(array=w394, index (col)=w389) -> (element=w391:i16[])  [unwired: 1 in]
                      n187 = Add(x=w391, y=w390) -> (x+y=w392:i32[])
                      n188 = Replace Array Subset(array=w390, new element=w392) -> (w393:i32[])  [unwired: 1 in]
                    }
                    n189 = Array Max & Min(array=w383) -> (max index (indices)=w382:i32)  [unwired: 3 out]
                  }
                  frame #2 {
                    n190 = property on="Zoom Window" class="IntGraph (strict)"() -> ("Y Scale.Range:Minimum"=w400:dbl)  [unwired: 2 in, 2 out]
                    n191 = property on="Zoom Window" class="IntGraph (strict)"() -> ("X Scale.Range:Maximum"=w402:dbl)  [unwired: 2 in, 2 out]
                    n192 = property on="Zoom Window" class="IntGraph (strict)"() -> ("X Scale.Range:Minimum"=w403:dbl)  [unwired: 2 in, 2 out]
                    n193 = property on="Zoom Window" class="IntGraph (strict)"() -> ("Y Scale.Range:Maximum"=w401:dbl)  [unwired: 2 in, 2 out]
                    n194 = Subtract(x=w401, y=w400) -> (x-y=w406:dbl)
                    n195 = Subtract(x=w402, y=w403) -> (x-y=w405:dbl)
                    n196 = Bundle(w405, w406) -> (w409:cluster{dbl, dbl})  [unwired: 1 in]
                    n197 = local read "X"() -> (w413:dbl)
                    n198 = local read "Y"() -> (w412:dbl)
                    n199 = Divide(x=w409, y=2) -> (x/y=w404:cluster{dbl, dbl})
                    n200 = Bundle(w408, w407) -> (w411:cluster{i32, i32})  [unwired: 1 in]
                    n201 = Bundle("X"=w413, "Y"=w412) -> (w410:cluster{"X":dbl, "Y":dbl})  [unwired: 1 in]
                    n202 = Subtract(x=w411, y=w404) -> (x-y=w398:cluster{dbl, dbl})
                    n203 = To Word Integer(number=w398) -> (16bit integer=w399:cluster{i16, i16})
                    n204 = To Double Precision Float(number=w399) -> (double precision float=w397:cluster{dbl, dbl})
                    n205 = Add(x=w397, y=w410) -> (x+y=w396:cluster{dbl, dbl})
                    n206 = To Word Integer(number=w396) -> (16bit integer=w395:cluster{i16, i16})
                  }
                  frame #3 {
                    n207 = local read "Image Display Resolution"() -> (w426:u16)
                    n208 = Enqueue Element(queue=w418, element=T5 {"Command"="ZOOM_FOR_GAUSS_FIT", "Parameter"=""}, error in (no error)=w417) -> (queue out=w415:refnum<queue>, error out=w416:errorcluster)  [unwired: 1 in, 1 out]
                    n209 = local read "Resolution Factor"() -> (w429:u16)
                    n210 = Enqueue Element(queue=w415, element=T5 {"Command"="FIT_GAUSSIAN", "Parameter"=""}, error in (no error)=w416) -> ()  [unwired: 1 in, 3 out]
                    n211 = Multiply(x=w426, y=w429) -> (x*y=w427:u16)
                    n212 = Equal To 0?(x=w426) -> (x = 0?=w424:bool)
                    n213 = Select(t=u16 1, s=w424, f=w427) -> (s? t:f=w428:u16)
                    n214 = To Double Precision Float(number=w428) -> (double precision float=w423:dbl)
                    n215 = Divide(x=w422, y=w423) -> (x/y=w421:cluster{dbl, dbl})
                    n216 = property on="Image" class="IntGraph (strict)"("Cursor.Cursor Position"=w421) -> ()  [unwired: 2 in, 2 out]
                  }
                }
              }
              frame 97 {
                n217 = local read "Zoom Window"() -> (w432:i16[][])
                n218 = Array Size(array=w432) -> (size(s)=w436:i32[])
                n219 = Index Array(array=w436, index=1) -> (element=w437:i32)
                n220 = Index Array(array=w436, index=0) -> (element=w434:i32)
                n221 = stacked-sequence {
                  seq-local: [w440 _ _] -> [_ w453 _]
                  seq-local: [_ w456 _] -> [_ _ w464]
                  tunnel: w432 -> [w444 _ _]
                  tunnel: w434 -> [w438 _ _]
                  tunnel: w437 -> [w439 _ _]
                  tunnel: w431 -> [_ _ w461]
                  tunnel: w430 -> [_ _ w462]
                  frame #0 {
                    n222 = Initialize Array(0 ("element"), w438) -> (w443:i32[])
                    n223 = for {
                      N: w439 -> [_]
                      tunnel: w444 -> [w450]
                      shift-right: [w449] -> w441
                      shift-left: w443 -> [w447]
                      i -> [w445]
                      n224 = Index Array(array=w450, index (col)=w445) -> (element=w448:i16[])  [unwired: 1 in]
                      n225 = Add(x=w448, y=w447) -> (x+y=w446:i32[])
                      n226 = Replace Array Subset(array=w447, new element=w446) -> (w449:i32[])  [unwired: 1 in]
                    }
                    n227 = Array Max & Min(array=w441) -> (max index (indices)=w440:i32)  [unwired: 3 out]
                  }
                  frame #1 {
                    n228 = property on="Zoom Window" class="IntGraph (strict)"() -> ("X Scale.Range:Minimum"=w454:dbl)  [unwired: 2 in, 2 out]
                    n229 = property on="Zoom Window" class="IntGraph (strict)"() -> ("X Scale.Range:Maximum"=w455:dbl)  [unwired: 2 in, 2 out]
                    n230 = Subtract(x=w455, y=w454) -> (x-y=w452:dbl)
                    n231 = Divide(x=w452, y=2) -> (x/y=w458:dbl)
                    n232 = local read "X"() -> (w451:dbl)
                    n233 = Subtract(x=w453, y=w458) -> (x-y=w457:dbl)
                    n234 = Add(x=w457, y=w451) -> (x+y=w456:dbl)
                  }
                  frame #2 {
                    n235 = local read "Image Display Resolution"() -> (w468:u16)
                    n236 = local read "Resolution Factor"() -> (w471:u16)
                    n237 = Enqueue Element(queue=w461, element=T5 {"Command"="UPDATE_ZOOM", "Parameter"=""}, error in (no error)=w462) -> ()  [unwired: 1 in, 3 out]
                    n238 = Multiply(x=w468, y=w471) -> (x*y=w469:u16)
                    n239 = Equal To 0?(x=w468) -> (x = 0?=w466:bool)
                    n240 = Select(t=u16 1, s=w466, f=w469) -> (s? t:f=w470:u16)
                    n241 = To Double Precision Float(number=w470) -> (double precision float=w465:dbl)
                    n242 = Divide(x=w464, y=w465) -> (x/y=w460:dbl)
                    n243 = property on="Image" class="IntGraph (strict)"("Cursor.Cursor Position:Cursor X"=w460) -> ()  [unwired: 2 in, 2 out]
                  }
                }
              }
              frame 116 {
                n244 = local write "Tab Control"(T4."Imaging" ("Tab Control")) -> ()
              }
              frame 115 {
                n245 = local read "Image Display Resolution"() -> (w482:u16)
                n246 = property on="Image" class="IntGraph (strict)"() -> ("Cursor.Cursor Position:Cursor Y"=w477:dbl)  [unwired: 2 in, 2 out]
                n247 = Enqueue Element(queue=w489, element=T5 {"Command"="BUILD_SPATIAL_CUT", "Parameter"=""}, error in (no error)=w490) -> (queue out=w486:refnum<queue>, error out=w487:errorcluster)  [unwired: 1 in, 1 out]
                n248 = Multiply(x=w482, y=u16 4) -> (x*y=w483:u16)
                n249 = Equal To 0?(x=w482) -> (x = 0?=w480:bool)
                n250 = Select(t=u16 1, s=w480, f=w483) -> (s? t:f=w484:u16)
                n251 = To Double Precision Float(number=w484) -> (double precision float=w478:dbl)
                n252 = local write "Tab Control"(T4."Spectroscopy" ("Tab Control")) -> ()
                n253 = Multiply(x=w477, y=w478) -> (x*y=w476:dbl)
                n254 = Enqueue Element(queue=w486, element=T5 {"Command"="BUILD_SPECTRUM", "Parameter"=""}, error in (no error)=w487) -> (queue out=w473:refnum<queue>, error out=w474:errorcluster)  [unwired: 1 in, 1 out]
                n255 = local write "Column Cut Cursor Position"(w476) -> ()
                n256 = Enqueue Element(queue=w473, element=T5 {"Command"="COMPUTE_WAVELENGTHS", "Parameter"=""}, error in (no error)=w474) -> ()  [unwired: 1 in, 3 out]
              }
              frame 99 {
                n257 = property on="Image" class="IntGraph (strict)"() -> ("X Scale.Range:Maximum"=w498:dbl)  [unwired: 2 in, 2 out]
                n258 = property on="Image" class="IntGraph (strict)"() -> ("Y Scale.Range:Maximum"=w500:dbl)  [unwired: 2 in, 2 out]
                n259 = property on="Image" class="IntGraph (strict)"() -> ("Y Scale.Range:Minimum"=w499:dbl)  [unwired: 2 in, 2 out]
                n260 = property on="Image" class="IntGraph (strict)"() -> ("X Scale.Range:Minimum"=w497:dbl)  [unwired: 2 in, 2 out]
                n261 = Subtract(x=w498, y=w497) -> (x-y=w496:dbl)
                n262 = Subtract(x=w500, y=w499) -> (x-y=w495:dbl)
                n263 = Bundle(w496, w495) -> (w494:cluster{dbl, dbl})  [unwired: 1 in]
                n264 = Divide(x=w494, y=2) -> (x/y=w492:cluster{dbl, dbl})
                n265 = property on="Image" class="IntGraph (strict)"("Cursor.Cursor Position"=w492) -> ()  [unwired: 2 in, 2 out]
              }
            }
          }
          event "Send Target Offset Position": Value Change {
            w507 = " " ("string")
            n266 = event-data() -> ()  [unwired: 1 in, 1 out]
            n267 = local read "X"() -> (w515:dbl)
            n268 = local read "Y"() -> (w514:dbl)
            n269 = Format Into String(w515) -> (resulting string=w513:string)  [unwired: 3 in, 1 out]
            n270 = Format Into String(w514) -> (resulting string=w512:string)  [unwired: 3 in, 1 out]
            n271 = Concatenate Strings("T" ("string"), w507, w513, w507, w512) -> (w510:string)
            n272 = Bundle("Command"="ACCEPT_OFFSET_COORD", w510) -> (w502:cluster{"Command":string, string})  [unwired: 1 in]
            n273 = Obtain Queue(name (unnamed)="SICAMERA_Command_Q", element data type=T5 {"Command"="", "Parameter"=""} ("element")) -> (queue out=w505:refnum<queue>, created new?=w504:bool, error out=w503:errorcluster)  [unwired: 3 in]
            n274 = case shown="False" w504 {
              tunnel: w502 -> [_ w523]
              tunnel: w505 -> [_ w522]
              tunnel: w503 -> [_ w521]
              tunnel: ["Error upon sending the offset coord." ("Image Status") "Coordinates successfully uploaded to GSCS!" ("Image Status")] -> w501
              frame True {
              }
              frame False {
                n275 = Enqueue Element(queue=w522, element=w523, error in (no error)=w521) -> (queue out=w520:refnum<queue>, error out=w519:errorcluster)  [unwired: 1 in, 1 out]
                n276 = Release Queue(queue=w520, error in (no error)=w519) -> ()  [unwired: 1 in, 3 out]
              }
            }
            n277 = local write "Send Target Offset Position"(FALSE ("Send Target Offset Position")) -> ()
            n278 = local write "Image Status"(w501) -> ()
          }
          event "Send Object Offset Position": Value Change {
            w527 = " " ("string")
            n279 = event-data() -> ()  [unwired: 1 in, 1 out]
            n280 = local read "X"() -> (w539:dbl)
            n281 = local read "Y"() -> (w538:dbl)
            n282 = Format Into String(w539) -> (resulting string=w537:string)  [unwired: 3 in, 1 out]
            n283 = Format Into String(w538) -> (resulting string=w536:string)  [unwired: 3 in, 1 out]
            n284 = Concatenate Strings("O" ("string"), w527, w537, w527, w536) -> (w534:string)
            n285 = Obtain Queue(name (unnamed)="SICAMERA_Command_Q", element data type=T5 {"Command"="", "Parameter"=""} ("element")) -> (queue out=w532:refnum<queue>, created new?=w525:bool, error out=w531:errorcluster)  [unwired: 3 in]
            n286 = Bundle("Command"="ACCEPT_OFFSET_COORD", w534) -> (w533:cluster{"Command":string, string})  [unwired: 1 in]
            n287 = case shown="True" w525 {
              tunnel: w533 -> [_ w546]
              tunnel: w532 -> [_ w545]
              tunnel: w531 -> [_ w544]
              tunnel: ["Error upon sending the offset coord." ("Image Status") "Coordinates successfully uploaded to GSCS!" ("Image Status")] -> w524
              frame True {
              }
              frame False {
                n288 = Enqueue Element(queue=w545, element=w546, error in (no error)=w544) -> (queue out=w543:refnum<queue>, error out=w542:errorcluster)  [unwired: 1 in, 1 out]
                n289 = Release Queue(queue=w543, error in (no error)=w542) -> ()  [unwired: 1 in, 3 out]
              }
            }
            n290 = local write "Send Object Offset Position"(FALSE ("Send Object Offset Position")) -> ()
            n291 = local write "Image Status"(w524) -> ()
          }
          event "Zoom In": Mouse Down {
            n292 = event-data() -> ()  [unwired: 1 in, 8 out]
            n293 = property on="Image" class="IntGraph (strict)"() -> ("X Scale.Range"=w566:T9)  [unwired: 2 in, 2 out]
            n294 = property on="Image" class="IntGraph (strict)"() -> ("Y Scale.Range"=w565:T9)  [unwired: 2 in, 2 out]
            n295 = Unbundle By Name(w566) -> ("Maximum"=w564:dbl, "Minimum"=w558:dbl)
            n296 = Unbundle By Name(w565) -> ("Maximum"=w557:dbl, "Minimum"=w547:dbl)
            n297 = Subtract(x=w564, y=w558) -> (x-y=w563:dbl)
            n298 = Subtract(x=w557, y=w547) -> (x-y=w562:dbl)
            n299 = Bundle(w563, w562) -> (w559:cluster{dbl, dbl})  [unwired: 1 in]
            n300 = Bundle("Minimum"=w558, "Minimum"=w547) -> (w555:cluster{"Minimum":dbl, "Minimum":dbl})  [unwired: 1 in]
            n301 = Multiply(x=w559, y=0.5) -> (x*y=w553:cluster{dbl, dbl})
            n302 = Multiply(x=w559, y=0.25) -> (x*y=w556:cluster{dbl, dbl})
            n303 = Add(x=w556, y=w555) -> (x+y=w554:cluster{dbl, dbl})
            n304 = Add(x=w553, y=w554) -> (x+y=w550:cluster{dbl, dbl})
            n305 = Unbundle(w554) -> (w552:dbl, w551:dbl)
            n306 = Unbundle(w550) -> (w549:dbl, w548:dbl)
            n307 = property on="Image" class="IntGraph (strict)"("Y Scale.Range:Minimum"=w551) -> ()  [unwired: 2 in, 2 out]
            n308 = property on="Image" class="IntGraph (strict)"("X Scale.Range:Minimum"=w552) -> ()  [unwired: 2 in, 2 out]
            n309 = property on="Image" class="IntGraph (strict)"("X Scale.Range:Maximum"=w549) -> ()  [unwired: 2 in, 2 out]
            n310 = property on="Image" class="IntGraph (strict)"("Y Scale.Range:Maximum"=w548) -> ()  [unwired: 2 in, 2 out]
          }
          event "Zoom Out": Mouse Down {
            n311 = event-data() -> ()  [unwired: 1 in, 8 out]
            n312 = property on="Image" class="IntGraph (strict)"() -> ("X Scale.Range"=w586:T9)  [unwired: 2 in, 2 out]
            n313 = property on="Image" class="IntGraph (strict)"() -> ("Y Scale.Range"=w585:T9)  [unwired: 2 in, 2 out]
            n314 = Unbundle By Name(w586) -> ("Maximum"=w584:dbl, "Minimum"=w578:dbl)
            n315 = Unbundle By Name(w585) -> ("Maximum"=w577:dbl, "Minimum"=w570:dbl)
            n316 = Subtract(x=w584, y=w578) -> (x-y=w583:dbl)
            n317 = Subtract(x=w577, y=w570) -> (x-y=w582:dbl)
            n318 = Bundle(w583, w582) -> (w579:cluster{dbl, dbl})  [unwired: 1 in]
            n319 = Bundle("Minimum"=w578, "Minimum"=w570) -> (w568:cluster{"Minimum":dbl, "Minimum":dbl})  [unwired: 1 in]
            n320 = Multiply(x=w579, y=2) -> (x*y=w569:cluster{dbl, dbl})
            n321 = Multiply(x=w569, y=0.25) -> (x*y=w567:cluster{dbl, dbl})
            n322 = Subtract(x=w568, y=w567) -> (x-y=w576:cluster{dbl, dbl})
            n323 = Add(x=w569, y=w576) -> (x+y=w573:cluster{dbl, dbl})
            n324 = Unbundle(w576) -> (w575:dbl, w574:dbl)
            n325 = Unbundle(w573) -> (w572:dbl, w571:dbl)
            n326 = property on="Image" class="IntGraph (strict)"("Y Scale.Range:Minimum"=w574) -> ()  [unwired: 2 in, 2 out]
            n327 = property on="Image" class="IntGraph (strict)"("X Scale.Range:Minimum"=w575) -> ()  [unwired: 2 in, 2 out]
            n328 = property on="Image" class="IntGraph (strict)"("X Scale.Range:Maximum"=w572) -> ()  [unwired: 2 in, 2 out]
            n329 = property on="Image" class="IntGraph (strict)"("Y Scale.Range:Maximum"=w571) -> ()  [unwired: 2 in, 2 out]
          }
          event "Refresh Spatial Cut": Value Change {
            n330 = event-data() -> ()  [unwired: 1 in, 6 out]
            n331 = Enqueue Element(queue=w587, element=T5 {"Command"="BUILD_SPATIAL_CUT", "Parameter"=""}, error in (no error)=w588) -> ()  [unwired: 1 in, 3 out]
          }
          event "Cut Along Column": Mouse Up {
            # "Remove rest of code (left) if not allowing clicking to create spectrum"
            n332 = event-data() -> ("Coords"=w608:T10)  [unwired: 1 in]
            n333 = Enqueue Element(queue=w596, element=T5 {"Command"="BUILD_SPECTRUM", "Parameter"=""}, error in (no error)=w598) -> (queue out=w595:refnum<queue>, error out=w597:errorcluster)  [unwired: 1 in, 1 out]
            n334 = Unbundle By Name(w608) -> ("Horizontal"=w607:i32)
            n335 = property on="Cut Along Column" class="WFGraph (strict)"() -> ("Plot Area:Size:Width"=w591:u32)  [unwired: 2 in, 2 out]
            n336 = property on="Cut Along Column" class="WFGraph (strict)"() -> ("X Scale.Position:Left"=w594:i32)  [unwired: 2 in, 2 out]
            n337 = Enqueue Element(queue=w595, element=T5 {"Command"="COMPUTE_WAVELENGTHS", "Parameter"=""}, error in (no error)=w597) -> ()  [unwired: 1 in, 3 out]
            n338 = Add(x=w594, y=9) -> (x+y=w592:i32)
            n339 = property on="Cut Along Column" class="WFGraph (strict)"() -> ("X Scale.Range:Maximum"=w604:dbl)  [unwired: 2 in, 2 out]
            n340 = property on="Cut Along Column" class="WFGraph (strict)"() -> ("X Scale.Range:Minimum"=w601:dbl)  [unwired: 2 in, 2 out]
            n341 = Subtract(x=w607, y=w592) -> (x-y=w606:i32)
            n342 = Subtract(x=w604, y=w601) -> (x-y=w603:dbl)
            n343 = Divide(x=w606, y=w591) -> (x/y=w605:dbl)
            n344 = property on="Cut Along Column" class="WFGraph (strict)"() -> ("Cursor.Cursor Position:Cursor X"=→"Column Cut Cursor Position":dbl)  [unwired: 2 in, 2 out]
            n345 = Multiply(x=w605, y=w603) -> (x*y=w602:dbl)
            n346 = Add(x=w602, y=w601) -> ()  [unwired: 1 out]
          }
          event "Refresh Spectrum": Value Change {
            n347 = event-data() -> ()  [unwired: 1 in, 6 out]
            n348 = Enqueue Element(queue=w613, element=T5 {"Command"="BUILD_SPECTRUM", "Parameter"=""}, error in (no error)=w612) -> (queue out=w609:refnum<queue>, error out=w610:errorcluster)  [unwired: 1 in, 1 out]
            n349 = Enqueue Element(queue=w609, element=T5 {"Command"="COMPUTE_WAVELENGTHS", "Parameter"=""}, error in (no error)=w610) -> ()  [unwired: 1 in, 3 out]
          }
          event "Show x scale in:": Value Change {
            n350 = event-data() -> ()  [unwired: 1 in, 1 out]
            n351 = Enqueue Element(queue=w615, element=T5 {"Command"="COMPUTE_WAVELENGTHS", "Parameter"=""}, error in (no error)=w616) -> ()  [unwired: 1 in, 3 out]
          }
          event "Image": Mouse Down {
            n352 = event-data() -> ("Coords"=w621:T10)  [unwired: 1 in, 3 out]
            n353 = stacked-sequence {
              tunnel: w621 -> [w642 _]
              tunnel: w620 -> [_ _]
              tunnel: w619 -> [_ w644]
              tunnel: w618 -> [_ w643]
              frame #0 {
                # "Useless code.  Get rid of if keeping reading of coordinates  by cursor."
                n354 = Unbundle By Name(w642) -> ("Horizontal"=w641:i32, "Vertical"=w633:i32)
                n355 = property on="Image" class="IntGraph (strict)"() -> ("X Scale.Position:Left"=w626:i32)  [unwired: 2 in, 2 out]
                n356 = property on="Image" class="IntGraph (strict)"() -> ("Y Scale.Position:Top"=w624:i32)  [unwired: 2 in, 2 out]
                n357 = property on="Image" class="IntGraph (strict)"() -> ("Y Scale.Bounds:Area Height"=w625:u32)  [unwired: 2 in, 2 out]
                n358 = property on="Image" class="IntGraph (strict)"() -> ("Y Scale.Range:Maximum"=w628:dbl)  [unwired: 2 in, 2 out]
                n359 = property on="Image" class="IntGraph (strict)"() -> ("Y Scale.Range:Minimum"=w629:dbl)  [unwired: 2 in, 2 out]
                n360 = property on="Image" class="IntGraph (strict)"() -> ("X Scale.Bounds:Area Width"=w632:u32)  [unwired: 2 in, 2 out]
                n361 = property on="Image" class="IntGraph (strict)"() -> ("X Scale.Range:Minimum"=w630:dbl)  [unwired: 2 in, 2 out]
                n362 = property on="Image" class="IntGraph (strict)"() -> ("X Scale.Range:Maximum"=w631:dbl)  [unwired: 2 in, 2 out]
                n363 = Subtract(x=w641, y=w626) -> (x-y=w640:i32)
                n364 = Subtract(x=w633, y=w624) -> (x-y=w634:i32)
                n365 = Divide(x=w640, y=w632) -> (x/y=w638:dbl)
                n366 = Divide(x=w634, y=w625) -> (x/y=w635:dbl)
                n367 = Subtract(x=w631, y=w630) -> (x-y=w639:dbl)
                n368 = Subtract(x=w628, y=w629) -> (x-y=w636:dbl)
                n369 = Multiply(x=w638, y=w639) -> (x*y=w637:dbl)
                n370 = Multiply(x=w635, y=w636) -> (x*y=w627:dbl)
                n371 = Add(x=w637, y=w630) -> (x+y=w623:dbl)
                n372 = property on="Image" class="IntGraph (strict)"("Cursor.Cursor Position:Cursor X"=w623) -> ()  [unwired: 2 in, 2 out]
                n373 = Subtract(x=w628, y=w627) -> (x-y=w622:dbl)
                n374 = property on="Image" class="IntGraph (strict)"("Cursor.Cursor Position:Cursor Y"=w622) -> ()  [unwired: 2 in, 2 out]
              }
              frame #1 {
                n375 = Enqueue Element(queue=w643, element=T5 {"Command"="UPDATE_ZOOM", "Parameter"=""}, error in (no error)=w644) -> ()  [unwired: 1 in, 3 out]
              }
            }
          }
          event "Cut Along Column": Mouse Enter {
            n376 = event-data() -> ()  [unwired: 1 in, 4 out]
            n377 = local write "Spectrum Status"("Click to create aperture and corresponding spectrum" ("Spectrum Status")) -> ()
          }
          event "Image Scale Stretch": Mouse Up {
            n378 = event-data() -> ()  [unwired: 1 in, 9 out]
            n379 = Enqueue Element(queue=w648, element=T5 {"Command"="SCALE_IMAGE", "Parameter"=""}, error in (no error)=w647) -> ()  [unwired: 1 in, 3 out]
          }
        }
      }
      frame "FIT_GAUSSIAN" {
        n380 = Multiply(x=w651, y=0.15) -> (x*y=w655:T2)
        n381 = local read "Zoom Window"() -> (w671:i16[][])
        n382 = Array Size(array=w671) -> (size(s)=w667:i32[])
        n383 = Unbundle By Name(w655) -> ("Serial Binning"=w657:dbl, "Parallel Binning"=w656:dbl)
        n384 = Index Array(array=w667, index=1) -> (element=w666:i32)
        n385 = Index Array(array=w667, index=0) -> (element=w669:i32)
        n386 = stacked-sequence {
          seq-local: [w673 _ _ _] -> [_ _ w713 _]
          seq-local: [_ w689 _ _] -> [_ _ w714 _]
          seq-local: [_ _ w705 _] -> [_ _ _ w726]
          tunnel: w671 -> [w682 w696 _ _]
          tunnel: w669 -> [w679 w695 _ _]
          tunnel: w666 -> [w678 w694 _ _]
          tunnel: w653 -> [_ _ _ w723]
          tunnel: w652 -> [_ _ _ w724]
          tunnel: [w675 _ _ _] -> w665
          tunnel: [_ w691 _ _] -> w664
          tunnel: w657 -> [w674 _ _ _]
          tunnel: w656 -> [_ w690 _ _]
          frame #0 {
            n387 = Initialize Array(0 ("element"), w678) -> (w681:i32[])
            n388 = for {
              N: w679 -> [_]
              tunnel: w682 -> [w688]
              shift-right: [w687] -> w677
              shift-left: w681 -> [w685]
              i -> [w683]
              n389 = Index Array(array=w688, index (row)=w683) -> (element=w686:i16[])  [unwired: 1 in]
              n390 = Add(x=w686, y=w685) -> (x+y=w684:i32[])
              n391 = Replace Array Subset(array=w685, new element=w684) -> (w687:i32[])  [unwired: 1 in]
            }
            n392 = call "Fit_1D_Gaussian.vi"("Input 1D Array"=w677) -> ("center"=w673:dbl, "FWHM"=w676:dbl)  [unwired: 3 in]
            n393 = Multiply(x=w676, y=w674) -> (x*y=w675:dbl)
          }
          frame #1 {
            n394 = Initialize Array(0 ("element"), w695) -> (w698:i32[])
            n395 = for {
              N: w694 -> [_]
              tunnel: w696 -> [w704]
              shift-right: [w703] -> w693
              shift-left: w698 -> [w700]
              i -> [w699]
              n396 = Index Array(array=w704, index (col)=w699) -> (element=w701:i16[])  [unwired: 1 in]
              n397 = Add(x=w701, y=w700) -> (x+y=w702:i32[])
              n398 = Replace Array Subset(array=w700, new element=w702) -> (w703:i32[])  [unwired: 1 in]
            }
            n399 = call "Fit_1D_Gaussian.vi"("Input 1D Array"=w693) -> ("center"=w689:dbl, "FWHM"=w692:dbl)  [unwired: 3 in]
            n400 = Multiply(x=w692, y=w690) -> (x*y=w691:dbl)
          }
          frame #2 {
            n401 = property on="Zoom Window" class="IntGraph (strict)"() -> ("X Scale.Range:Maximum"=w712:dbl)  [unwired: 2 in, 2 out]
            n402 = property on="Zoom Window" class="IntGraph (strict)"() -> ("X Scale.Range:Minimum"=w711:dbl)  [unwired: 2 in, 2 out]
            n403 = property on="Zoom Window" class="IntGraph (strict)"() -> ("Y Scale.Range:Maximum"=w710:dbl)  [unwired: 2 in, 2 out]
            n404 = property on="Zoom Window" class="IntGraph (strict)"() -> ("Y Scale.Range:Minimum"=w709:dbl)  [unwired: 2 in, 2 out]
            n405 = Subtract(x=w710, y=w709) -> (x-y=w708:dbl)
            n406 = Subtract(x=w712, y=w711) -> (x-y=w707:dbl)
            n407 = Bundle(w707, w708) -> (w715:cluster{dbl, dbl})  [unwired: 1 in]
            n408 = local read "X"() -> (w720:dbl)
            n409 = local read "Y"() -> (w719:dbl)
            n410 = Divide(x=w715, y=2) -> (x/y=w706:cluster{dbl, dbl})
            n411 = Bundle("center"=w714, "center"=w713) -> (w718:cluster{"center":dbl, "center":dbl})  [unwired: 1 in]
            n412 = Bundle("X"=w720, "Y"=w719) -> (w717:cluster{"X":dbl, "Y":dbl})  [unwired: 1 in]
            n413 = Subtract(x=w718, y=w706) -> (x-y=w716:cluster{dbl, dbl})
            n414 = Add(x=w716, y=w717) -> (x+y=w705:cluster{dbl, dbl})
          }
          frame #3 {
            n415 = local read "Image Display Resolution"() -> (w730:u16)
            n416 = local read "Resolution Factor"() -> (w733:u16)
            n417 = Enqueue Element(queue=w723, element=T5 {"Command"="UPDATE_ZOOM", "Parameter"=""}, error in (no error)=w724) -> ()  [unwired: 1 in, 3 out]
            n418 = Multiply(x=w730, y=w733) -> (x*y=w731:u16)
            n419 = Equal To 0?(x=w730) -> (x = 0?=w728:bool)
            n420 = Select(t=u16 1, s=w728, f=w731) -> (s? t:f=w732:u16)
            n421 = To Double Precision Float(number=w732) -> (double precision float=w727:dbl)
            n422 = Divide(x=w726, y=w727) -> (x/y=w722:cluster{dbl, dbl})
            n423 = property on="Image" class="IntGraph (strict)"("Cursor.Cursor Position"=w722) -> ()  [unwired: 2 in, 2 out]
          }
        }
        n424 = Add(x=w665, y=w664) -> (x+y=w663:dbl)
        n425 = Divide(x=w663, y=2.0) -> (x/y=w661:dbl)
        n426 = Format Into String(format string="%.1f", w661) -> (resulting string=w672:string)  [unwired: 2 in, 1 out]
        n427 = Concatenate Strings("Star centered; FWHM is ~" ("Image Status"), w672, " \"" ("string")) -> (w659:string)
        n428 = local write "Image Status"(w659) -> ()
      }
      frame "SCALE_IMAGE" {
        n429 = local read "Image"() -> (w743:dbl[][])
        n430 = property on="Zoom Window" class="IntGraph (strict)"("Z Scale.Mapping Mode"=u8 1) -> ()  [unwired: 2 in, 2 out]
        n431 = Array Max & Min(array=w743) -> (max value=w738:dbl)  [unwired: 3 out]
        n432 = Array Size(array=w743) -> (size(s)=w742:i32[])
        n433 = Multiply Array Elements(1:w742) -> (0:w740:i32)
        n434 = Divide(x="Image Scale Stretch", y=500.0) -> (x/y=w746:cluster{dbl, dbl})
        n435 = Add Array Elements(numeric array=w743) -> (sum=w741:dbl)
        n436 = Divide(x=w741, y=w740) -> (x/y=w739:dbl)
        n437 = Multiply(x=w746, y=w738) -> (x*y=w745:cluster{dbl, dbl})
        n438 = local write "Image Status"("Re-scaling image..." ("Status")) -> ()
        n439 = Add(x=w745, y=w739) -> (x+y=w744:cluster{dbl, dbl})
        n440 = Unbundle(w744) -> (w736:dbl, w737:dbl)
        n441 = property on="Zoom Window" class="IntGraph (strict)"("Z Scale.Range:Minimum"=w736) -> ()  [unwired: 2 in, 2 out]
        n442 = property on="Image" class="IntGraph (strict)"("Z Scale.Range:Minimum"=w736) -> ()  [unwired: 2 in, 2 out]
        n443 = property on="Image" class="IntGraph (strict)"("Z Scale.Range:Maximum"=w737) -> ()  [unwired: 2 in, 2 out]
        n444 = property on="Zoom Window" class="IntGraph (strict)"("Z Scale.Range:Maximum"=w737) -> ()  [unwired: 2 in, 2 out]
      }
      frame "UPDATE_ZOOM" {
        n445 = local read "Image Display Resolution"() -> (w774:u16)
        n446 = local read "Resolution Factor"() -> (w767:u16)
        n447 = property on="Image" class="IntGraph (strict)"() -> ("Cursor.Cursor Position"=w772:T11)  [unwired: 2 in, 2 out]
        n448 = Multiply(x=w774, y=w767) -> (x*y=w773:u16)
        n449 = Equal To 0?(x=w774) -> (x = 0?=w776:bool)
        n450 = Select(t=u16 1, s=w776, f=w773) -> (s? t:f=w770:u16)
        n451 = To Double Precision Float(number=w770) -> (double precision float=w769:dbl)
        n452 = Multiply(x=w772, y=w769) -> (x*y=w771:T11)
        n453 = Unbundle(w771) -> ("Cursor X"=w768:dbl, "Cursor Y"=w778:dbl)
        "X" <- w768
        "Y" <- w778
        n454 = property on="Image" class="IntGraph (strict)"() -> ("Bounds:Area Width"=w763:u32)  [unwired: 2 in, 2 out]
        n455 = Index Array(array=w777, index (row)=w768, index (col)=w778) -> (element=→"Value":i16)
        n456 = Divide(x=w763, y="Zoom Window Width (1/x)") -> (x/y=w762:dbl)
        n457 = property on="Image" class="IntGraph (strict)"() -> ("Bounds:Area Height"=w758:u32)  [unwired: 2 in, 2 out]
        n458 = To Word Integer(number=w762) -> (16bit integer=w757:i16)
        n459 = Divide(x=w757, y=2.0) -> (x/y=w765:dbl)
        n460 = Divide(x=w758, y="Zoom Window Width (1/x)") -> (x/y=w759:dbl)
        n461 = To Word Integer(number=w765) -> (16bit integer=w764:i16)
        n462 = To Word Integer(number=w759) -> (16bit integer=w756:i16)
        n463 = Subtract(x=w768, y=w764) -> (x-y=w750:dbl)
        n464 = Divide(x=w756, y=2.0) -> (x/y=w760:dbl)
        n465 = To Word Integer(number=w760) -> (16bit integer=w755:i16)
        n466 = Subtract(x=w778, y=w755) -> (x-y=w752:dbl)
        n467 = To Word Integer(number=w750) -> (16bit integer=w749:i16)
        n468 = To Word Integer(number=w752) -> (16bit integer=w751:i16)
        n469 = Array Subset(array=w777, index (row)=w749, length (row)=w757, index (col)=w751, length (col)=w756) -> (→"Zoom Window":i16[][])
        n470 = Bundle(w764, w755) -> (w754:cluster{i16, i16})  [unwired: 1 in]
        n471 = property on="Zoom Window" class="IntGraph (strict)"("Cursor.Cursor Position"=w754) -> ()  [unwired: 2 in, 2 out]
      }
      frame "ZOOM_FOR_GAUSS_FIT" {
        n472 = local read "Image Display Resolution"() -> (w787:u16)
        n473 = local read "Resolution Factor"() -> (w792:u16)
        n474 = property on="Image" class="IntGraph (strict)"() -> ("Cursor.Cursor Position"=w784:T11)  [unwired: 2 in, 2 out]
        n475 = local read "Zoom Window Width (1/x)"() -> (w804:u32)
        n476 = Multiply(x=w787, y=w792) -> (x*y=w788:u16)
        n477 = Equal To 0?(x=w787) -> (x = 0?=w785:bool)
        n478 = Select(t=u16 1, s=w785, f=w788) -> (s? t:f=w790:u16)
        n479 = To Double Precision Float(number=w790) -> (double precision float=w791:dbl)
        n480 = property on="Image" class="IntGraph (strict)"() -> ("Bounds:Area Width"=w803:u32)  [unwired: 2 in, 2 out]
        n481 = Multiply(x=w784, y=w791) -> (x*y=w789:T11)
        n482 = Unbundle(w789) -> ("Cursor X"=w782:dbl, "Cursor Y"=w781:dbl)
        n483 = Divide(x=w803, y=w804) -> (x/y=w810:dbl)
        n484 = To Word Integer(number=w810) -> (16bit integer=w807:i16)
        n485 = local write "X"(w782) -> ()
        n486 = property on="Image" class="IntGraph (strict)"() -> ("Bounds:Area Height"=w802:u32)  [unwired: 2 in, 2 out]
        n487 = local write "Y"(w781) -> ()
        n488 = Divide(x=w807, y=2.0) -> (x/y=w796:dbl)
        n489 = Divide(x=w802, y=w804) -> (x/y=w808:dbl)
        n490 = To Word Integer(number=w796) -> (16bit integer=w794:i16)
        n491 = To Word Integer(number=w808) -> (16bit integer=w806:i16)
        n492 = Subtract(x=w782, y=w794) -> (x-y=w800:dbl)
        n493 = Divide(x=w806, y=2.0) -> (x/y=w795:dbl)
        n494 = To Word Integer(number=w800) -> (16bit integer=w799:i16)
        n495 = To Word Integer(number=w795) -> (16bit integer=w793:i16)
        n496 = Subtract(x=w781, y=w793) -> (x-y=w797:dbl)
        n497 = To Word Integer(number=w797) -> (16bit integer=w798:i16)
        n498 = Array Subset(array=w783, index (row)=w799, length (row)=w807, index (col)=w798, length (col)=w806) -> (w805:i16[][])
        n499 = Bundle(w794, w793) -> (w801:cluster{i16, i16})  [unwired: 1 in]
        n500 = property on="Zoom Window" class="IntGraph (strict)"("Cursor.Cursor Position"=w801) -> ()  [unwired: 2 in, 2 out]
        n501 = local write "Zoom Window"(w805) -> ()
      }
      frame "COMPUTE_WAVELENGTHS" {
        (unwired) dbl[][] [[0.0]]
        n502 = Unbundle By Name(w841) -> ("Camera Angle"=w814:dbl, "Grating Angle"=w813:dbl, "Grating"=w812:dbl, "Serial Origin"=w829:dbl, "Serial Binning"=w815:dbl)
        n503 = property on="Show x scale in:" class="LstBox (strict)"() -> ("Value"=w833:i32)  [unwired: 2 in, 2 out]
        n504 = local read "Raw Spectrum Array"() -> (w840:dbl[])
        n505 = Bundle("Camera Angle"=w814, "Grating Angle"=w813) -> (w847:cluster{"Camera Angle":dbl, "Grating Angle":dbl})  [unwired: 1 in]
        n506 = Divide(x=3.141592653589793, y=180.0) -> (x/y=w848:dbl)
        n507 = Equal?(x=w833, y=1) -> (x = y?=w837:bool)
        n508 = Multiply(x=w848, y=w847) -> (x*y=w846:cluster{"Camera Angle":dbl, "Grating Angle":dbl})
        n509 = Select(t=10000000.0, s=w837, f=1000000.0) -> (s? t:f=w834:dbl)
        n510 = Subtract(x=w829, y=140.0) -> (x-y=w831:dbl)
        n511 = Reciprocal(x=w812) -> (1/x=w843:dbl)
        n512 = Array Size(array=w840) -> (size(s)=w839:i32)
        n513 = Unbundle(w846) -> ("Camera Angle"=w845:dbl, "Grating Angle"=w844:dbl)
        n514 = Initialize Array(0.0 ("element"), w839) -> ()  [unwired: 1 out]
        n515 = Multiply(x=w843, y=w834) -> (x*y=w842:dbl)
        n516 = for {
          N: w839 -> [_]
          tunnel: w845 -> [w863]
          tunnel: w844 -> [w862]
          tunnel: w842 -> [w861]
          tunnel: w840 -> [w858] mode=indexing
          tunnel: w831 -> [w860]
          shift-right: [w853] -> w827
          shift-left: cluster{"x":dbl, "element":dbl}[] [] -> [w856]
          tunnel: w833 -> [w855]
          tunnel: w815 -> [w851]
          i -> [w852]
          n517 = case shown="1, 2" w855 {
            selector: w855 -> [_ w874]
            tunnel: w863 -> [_ w887]
            tunnel: w862 -> [_ w886]
            tunnel: w861 -> [_ w885]
            tunnel: w860 -> [_ w878]
            tunnel: [w865 w876] -> w857
            tunnel: w852 -> [w865 w875]
            tunnel: ["Pixel" ("X Scale.Name Label.Text") w871] -> w854
            tunnel: w851 -> [_ w867]
            frame 0, Default {
            }
            frame 1, 2 {
              # "camera focal length (mm)"
              # "middle pixel on chip"
              # "Plate scale (mm/pix)"
              n518 = Add(x=w878, y=w875) -> (x+y=w877:dbl)
              n519 = Divide(x=2048.0 ("y"), y=w867) -> (x/y=w866:dbl)
              n520 = Subtract(x=w877, y=w866) -> (x-y=w883:dbl)
              n521 = Equal?(x=w874, y=1) -> (x = y?=w872:bool)
              n522 = Multiply(x=0.015, y=w883) -> (x*y=w882:dbl)
              n523 = Divide(x=w882, y=366.0) -> (x/y=w880:dbl)
              n524 = Inverse Tangent(1:w880) -> (0:w879:dbl)
              n525 = formula code="x=L*(sin(a)+sin(b-a+delta));"("b"=w887, "a"=w886, "L"=w885, "delta"=w879) -> ("x"=w876:dbl)
              n526 = Select(t="Approiximate Wavelength (A)" ("X Scale.Name Label.Text"), s=w872, f="Approximate Wavelength (nm)" ("X Scale.Name Label.Text")) -> (s? t:f=w871:string)
            }
          }
          n527 = Bundle("x"=w857, "element"=w858) -> (w859:cluster{"x":dbl, "element":dbl})  [unwired: 1 in]
          n528 = Insert Into Array(array=w856, index=w852, new element=w859) -> (w853:cluster{"x":dbl, "element":dbl}[])
          n529 = property on="Calib Spec" class="XYGraph (strict)"("X Scale.Name Label.Text"=w854) -> ()  [unwired: 2 in, 2 out]
        }
        "Calib Spec" <- w827
        n530 = Array Max & Min(array=w827) -> (max value=w826:cluster{"x":dbl, "element":dbl}, min value=w825:cluster{"x":dbl, "element":dbl})  [unwired: 2 out]
        n531 = Unbundle(w826) -> ("x"=w821:dbl)  [unwired: 1 out]
        n532 = Unbundle(w825) -> ("x"=w820:dbl)  [unwired: 1 out]
        n533 = Subtract(x=w821, y=w820) -> (x-y=w824:dbl)
        n534 = Multiply(x=w824, y=0.02) -> (x*y=w822:dbl)
        n535 = Add(x=w820, y=w822) -> (x+y=w816:dbl)
        n536 = Subtract(x=w821, y=w822) -> (x-y=w817:dbl)
        n537 = To Word Integer(number=w816) -> (16bit integer=w819:i16)
        n538 = To Word Integer(number=w817) -> (16bit integer=w818:i16)
        n539 = property on="Calib Spec" class="XYGraph (strict)"("X Scale.Range:Minimum"=w819) -> ()  [unwired: 2 in, 2 out]
        n540 = property on="Calib Spec" class="XYGraph (strict)"("X Scale.Range:Maximum"=w818) -> ()  [unwired: 2 in, 2 out]
      }
      frame "DRAW_COMPASS" {
        w890 = T12 {"Font Name:"="", "Size"=14, "Strikeout?"=FALSE, "Italic?"=FALSE, "Underline?"=FALSE, "Outline?"=FALSE, "Shadow?"=FALSE, "Bold?"=TRUE} ("[user-specified font]")
        w912 = T13 {"horizontal"=enum."center", "vertical"=enum."center"} ("alignment(left, top)")
        w889 = T14."User-specified Font" ("desired font(Application)")
        w895 = 25
        w930 = u32 16448250 ("text color(black)")
        w899 = 50
        w947 = u32 16448250 ("text color(black)")
        w921 = 35
        w920 = 25
        n541 = Unbundle By Name(w909) -> ("Pos. Angle"=w888:dbl, "Azimuth"=w894:dbl)
        n542 = expression code="x*3.1415/180"(w894) -> (w893:dbl)
        n543 = expression code="x*3.1415/180"(w888) -> (w924:dbl)
        n544 = Add(x=1.5707963267948966, y=w924) -> (x+y=w908:dbl)
        n545 = Add(x=w908, y=w893) -> (x+y=w907:dbl)
        n546 = Sine(x=w908) -> (sin(x)=w911:dbl)
        n547 = Cosine(x=w908) -> (cos(x)=w910:dbl)
        n548 = Sine(x=w907) -> (sin(x)=w892:dbl)
        n549 = Cosine(x=w907) -> (cos(x)=w891:dbl)
        n550 = Sine(x=w924) -> (sin(x)=w923:dbl)
        n551 = Cosine(x=w924) -> (cos(x)=w925:dbl)
        n552 = Bundle(w925, w923) -> (w941:cluster{dbl, dbl})  [unwired: 1 in]
        n553 = Bundle(w910, w911) -> (w927:cluster{dbl, dbl})  [unwired: 1 in]
        n554 = Multiply(x=w920, y=w941) -> (x*y=w946:cluster{dbl, dbl})
        n555 = Multiply(x=w920, y=w941) -> (x*y=w943:cluster{dbl, dbl})
        n556 = Multiply(x=w921, y=w941) -> (x*y=w944:cluster{dbl, dbl})
        n557 = Multiply(x=w921, y=w941) -> (x*y=w940:cluster{dbl, dbl})
        n558 = Subtract(x=w899, y=w946) -> (x-y=w945:cluster{dbl, dbl})
        n559 = Add(x=w899, y=w943) -> (x+y=w942:cluster{dbl, dbl})
        n560 = Subtract(x=w899, y=w944) -> (x-y=w939:cluster{dbl, dbl})
        n561 = Multiply(x=w920, y=w927) -> (x*y=w929:cluster{dbl, dbl})
        n562 = Multiply(x=w920, y=w927) -> (x*y=w915:cluster{dbl, dbl})
        n563 = Multiply(x=w921, y=w927) -> (x*y=w918:cluster{dbl, dbl})
        n564 = Bundle(w891, w892) -> (w904:cluster{dbl, dbl})  [unwired: 1 in]
        n565 = Multiply(x=w921, y=w927) -> (x*y=w917:cluster{dbl, dbl})
        n566 = Add(x=w899, y=w940) -> (x+y=w938:cluster{dbl, dbl})
        n567 = call <vilib>:"Move Pen.vi"("new position"=w945, "picture"="Black Square") -> ("new picture"=w951:picture)  [unwired: 3 in]
        n568 = Add(x=w899, y=w929) -> (x+y=w928:cluster{dbl, dbl})
        n569 = Subtract(x=w899, y=w915) -> (x-y=w914:cluster{dbl, dbl})
        n570 = Subtract(x=w899, y=w918) -> (x-y=w926:cluster{dbl, dbl})
        n571 = Add(x=w899, y=w917) -> (x+y=w916:cluster{dbl, dbl})
        n572 = Multiply(x=w895, y=w904) -> (x*y=w902:cluster{dbl, dbl})
        n573 = call <vilib>:"Draw Line.vi"("picture"=w951, "end point"=w942, "color(black)"=u32 16448250, "pen"=T7 {"Width"=2, "Style"=enum."Solid"}) -> ("new picture"=w950:picture)  [unwired: 5 in]
        n574 = Multiply(x=w895, y=w904) -> (x*y=w905:cluster{dbl, dbl})
        n575 = Add(x=w899, y=w902) -> (x+y=w903:cluster{dbl, dbl})
        n576 = Subtract(x=w899, y=w905) -> (x-y=w906:cluster{dbl, dbl})
        n577 = call <vilib>:"Draw Text at Point.vi"("[user-specified font]"=w890, "text color(black)"=w947, "desired font(Application)"=w889, "text"="W", "alignment(left, top)"=w912, "origin"=w939, "picture"=w950) -> ("new picture"=w948:picture)  [unwired: 3 in, 1 out]
        n578 = call <vilib>:"Draw Text at Point.vi"("[user-specified font]"=w890, "text color(black)"=w947, "desired font(Application)"=w889, "text"="E", "alignment(left, top)"=w912, "origin"=w938, "picture"=w948) -> ("new picture"=w922:picture)  [unwired: 3 in, 1 out]
        n579 = call <vilib>:"Move Pen.vi"("new position"=w928, "picture"=w922) -> ("new picture"=w934:picture)  [unwired: 3 in]
        n580 = call <vilib>:"Draw Line.vi"("picture"=w934, "end point"=w914, "color(black)"=u32 16448250, "pen"=T7 {"Width"=2, "Style"=enum."Solid"}) -> ("new picture"=w933:picture)  [unwired: 5 in]
        n581 = call <vilib>:"Draw Text at Point.vi"("[user-specified font]"=w890, "text color(black)"=w930, "desired font(Application)"=w889, "text"="N", "alignment(left, top)"=w912, "origin"=w926, "picture"=w933) -> ("new picture"=w931:picture)  [unwired: 3 in, 1 out]
        n582 = call <vilib>:"Draw Text at Point.vi"("[user-specified font]"=w890, "text color(black)"=w930, "desired font(Application)"=w889, "text"="S", "alignment(left, top)"=w912, "origin"=w916, "picture"=w931) -> ("new picture"=w897:picture)  [unwired: 3 in, 1 out]
        n583 = call <vilib>:"Move Pen.vi"("new position"=w903, "picture"=w897) -> ("new picture"=w901:picture)  [unwired: 3 in]
        n584 = call <vilib>:"Draw Line.vi"("picture"=w901, "end point"=w906, "color(black)"=u32 16767232, "pen"=T7 {"Width"=2, "Style"=enum."Dash"}) -> ("new picture"=→"Compass":picture)  [unwired: 5 in]
      }
      frame "BUILD_SPATIAL_CUT" {
        n585 = Index Array(array=w964, index (row)="Cut Along Column #") -> (element=w957:i16[])  [unwired: 1 in]
        "Cut Along Column" <- w957
        n586 = Array Size(array=w957) -> (size(s)=w955:i32)
        n587 = Multiply(x=w955, y=0.02) -> (x*y=w962:dbl)
        n588 = Add(x=0.0, y=w962) -> (x+y=w960:dbl)
        n589 = Subtract(x=w955, y=w962) -> (x-y=w961:dbl)
        n590 = To Word Integer(number=w960) -> (16bit integer=w959:i16)
        n591 = To Word Integer(number=w961) -> (16bit integer=w958:i16)
        n592 = property on="Cut Along Column" class="WFGraph (strict)"("X Scale.Range:Minimum"=w959) -> ()  [unwired: 2 in, 2 out]
        n593 = property on="Cut Along Column" class="WFGraph (strict)"("X Scale.Range:Maximum"=w958) -> ()  [unwired: 2 in, 2 out]
      }
      frame "BUILD_SPECTRUM" {
        (unwired) i32[] array[4143 elements] ("Spectrum")
        n594 = local read "Column Cut Cursor Position"() -> (w966:dbl)
        n595 = Unbundle By Name(w971) -> ("# Columns (raw)"=w974:dbl)
        n596 = Quotient & Remainder(x="Aperture Width (pix)", y=2.0) -> (floor(x/y)=w978:dbl)  [unwired: 1 out]
        n597 = Subtract(x=w966, y=w978) -> (x-y=w977:dbl)
        n598 = property on="Cut Along Column" class="WFGraph (strict)"("Cursor.Cursor Position:Cursor X"=w966) -> ()  [unwired: 2 in, 2 out]
        n599 = Initialize Array(0.0 ("element"), w974) -> (w973:dbl[])
        n600 = for {
          N: "Aperture Width (pix)" -> [_]
          tunnel: w967 -> [w986]
          tunnel: w977 -> [w984]
          shift-right: [w982] -> w972
          shift-left: w973 -> [w981]
          i -> [w983]
          n601 = Add(x=w984, y=w983) -> (x+y=w985:dbl)
          n602 = Index Array(array=w986, index (col)=w985) -> (element=w980:i16[])  [unwired: 1 in]
          n603 = Add(x=w980, y=w981) -> (x+y=w982:dbl[])
        }
        "Raw Spectrum Array" <- w972
        n604 = Number To Decimal String(number=w966) -> (decimal integer string=w970:string)  [unwired: 1 in]
        n605 = Concatenate Strings("Spectrum Centered at Row " ("string"), w970) -> (w968:string)
        n606 = property on="Calib Spec" class="XYGraph (strict)"("Caption.Text"=w968) -> ()  [unwired: 2 in, 2 out]
      }
      frame "OPEN_FITS_FILE" {
        n607 = case shown="True" "Automatic Acquisition?" {
          tunnel: w990 -> [_ w998]
          tunnel: w989 -> [_ w995]
          tunnel: w988 -> [_ w992]
          frame False {
          }
          frame True {
            n608 = Concatenate Strings("", w992) -> ()  [unwired: 1 out]
            n609 = String To Path(string=w992) -> (path=w993:path)
            n610 = call "gfitsio-open-file.vi"("error in (no error)"=w998, "read only? (T:no)"=TRUE, "path"=w993) -> ("error out"=w996:errorcluster, "gfits refnum"=→"gfits refnum":T3)  [unwired: 7 in]
            n611 = case shown="No Error" w996 {
              selector: w996 -> [w1010 w1013]
              tunnel: w995 -> [w1009 _]
              tunnel: w992 -> [w1004 _]
              frame No Error {
                n612 = Enqueue Element(queue=w1009, element=T5 {"Command"="READ_FITS_HEADER", "Parameter"=""}, error in (no error)=w1010) -> (queue out=w1005:refnum<queue>, error out=w1006:errorcluster)  [unwired: 1 in, 1 out]
                n613 = property on="Image" class="IntGraph (strict)"("Caption.Text"=w1004) -> ()  [unwired: 2 in, 2 out]
                n614 = Enqueue Element(queue=w1005, element=T5 {"Command"="CONVERT_FITS_FILE", "Parameter"=""}, error in (no error)=w1006) -> (queue out=w1002:refnum<queue>, error out=w999:errorcluster)  [unwired: 1 in, 1 out]
                n615 = Enqueue Element(queue=w1002, element=T5 {"Command"="REPAIR_LOST_ROWS", "Parameter"=""}, error in (no error)=w999) -> (queue out=w1001:refnum<queue>, error out=w1000:errorcluster)  [unwired: 1 in, 1 out]
                n616 = Enqueue Element(queue=w1001, element=T5 {"Command"="DISPLAY_IMAGE", "Parameter"=""}, error in (no error)=w1000) -> ()  [unwired: 1 in, 3 out]
              }
              frame Error {
                n617 = One Button Dialog(message="ERROR:  Access to the FITS file could not be obtained.  Please ensure the server is properly cross-mounted to the storage disk. ") -> ()  [unwired: 1 in, 1 out]
                "error IO" <- w1013
              }
            }
          }
        }
      }
      frame "READ_FITS_HEADER" {
        # "PARAM16=Serial Origin\nPARAM20=Parallel Origin\nPARAM18=Serial Binning\nPARAM22=Parallel Binning"
        n618 = call "gfitsio-get-image-size.vi"("error in (no error)"=w1020, "gfits refnum"=w1021) -> ("naxes"=w1024:i32[], "dup gfits refnum"=w1019:T3)  [unwired: 6 in, 2 out]
        n619 = Index Array(array=w1024, index=1) -> (element=w1023:i32)
        n620 = Index Array(array=w1024, index=2) -> (element=w1022:i32)
        n621 = Bundle By Name(cluster=w1018, "# Rows (raw)"=w1023, "# Columns (raw)"=w1022) -> (w1015:T2)
        n622 = call "gfitsio-read-header.vi"("gfits refnum"=w1019) -> ("header"=w1014:string[])  [unwired: 8 in, 2 out]
        "FITS Header" <- w1014
        n623 = for {
          tunnel: string[] ["CAM_ANG", "PARAM20", "PARAM16", "GRT_ANG", "PARAM18", "PARAM22", "MOUNT_AZ", "PARAM21", "PARAM17", "POSANGLE", "GRATING"] -> [w1029]
          tunnel: w1014 -> [w1030] mode=indexing
          shift-right: [w1027] -> w1016
          shift-left: w1015 -> [w1028]
          n624 = for {
            tunnel: w1030 -> [w1033]
            tunnel: w1029 -> [w1035] mode=indexing
            shift-right: [w1032] -> w1027
            shift-left: w1028 -> [w1031]
            n625 = Match Pattern(string=w1033, regular expression=w1035) -> (after substring=w1034:string, offset past match=w1036:i32)  [unwired: 1 in, 2 out]
            n626 = Less Than 0?(x=w1036) -> (x < 0?=w1037:bool)
            n627 = case shown="False" w1037 {
              tunnel: w1035 -> [w1046 _]
              tunnel: w1031 -> [w1045 w1086]
              tunnel: w1034 -> [w1042 _]
              tunnel: [w1040 w1086] -> w1032
              frame False {
                n628 = Match Pattern(string=w1042, regular expression="=") -> (after substring=w1038:string)  [unwired: 1 in, 3 out]
                n629 = Match Pattern(string=w1038, regular expression="/") -> (before substring=w1039:string)  [unwired: 1 in, 3 out]
                n630 = Fract/Exp String To Number(string=w1039) -> (number=w1041:dbl)  [unwired: 3 in, 1 out]
                n631 = case shown="\"GRATING\"" w1046 {
                  tunnel: w1045 -> [w1047 w1049 w1052 w1055 w1058 w1062 w1063 w1071 w1074 w1078 w1082 w1084]
                  tunnel: w1041 -> [_ w1048 w1051 w1054 w1057 w1061 w1064 _ w1075 w1077 w1080 w1083]
                  tunnel: [w1047 w1050 w1053 w1056 w1059 w1060 w1065 w1070 w1076 w1079 w1081 w1085] -> w1040
                  tunnel: w1038 -> [_ _ _ _ _ _ _ w1072 _ _ _ _]
                  frame "", Default {
                  }
                  frame "PARAM16" {
                    n632 = Bundle By Name(cluster=w1049, "Serial Origin"=w1048) -> (w1050:T2)
                  }
                  frame "PARAM17" {
                    n633 = Bundle By Name(cluster=w1052, "Serial Length"=w1051, "# Columns (raw)"=w1051) -> (w1053:T2)
                  }
                  frame "PARAM18" {
                    n634 = Bundle By Name(cluster=w1055, "Serial Binning"=w1054) -> (w1056:T2)
                  }
                  frame "PARAM20" {
                    n635 = Bundle By Name(cluster=w1058, "Parallel Origin"=w1057) -> (w1059:T2)
                  }
                  frame "PARAM21" {
                    n636 = Bundle By Name(cluster=w1062, "Parallel Length"=w1061, "# Rows (raw)"=w1061) -> (w1060:T2)
                  }
                  frame "POSANGLE" {
                    n637 = Bundle By Name(cluster=w1063, "Pos. Angle"=w1064) -> (w1065:T2)
                  }
                  frame "GRATING" {
                    n638 = Match Pattern(string=w1072, regular expression="_") -> (after substring=w1067:string)  [unwired: 1 in, 3 out]
                    n639 = Match Pattern(string=w1067, regular expression="'") -> (before substring=w1066:string)  [unwired: 1 in, 3 out]
                    n640 = Fract/Exp String To Number(string=w1066) -> (number=w1069:dbl)  [unwired: 3 in, 1 out]
                    n641 = Bundle By Name(cluster=w1071, "Grating"=w1069) -> (w1070:T2)
                  }
                  frame "PARAM22" {
                    n642 = Bundle By Name(cluster=w1074, "Parallel Binning"=w1075) -> (w1076:T2)
                  }
                  frame "CAM_ANG" {
                    n643 = Bundle By Name(cluster=w1078, "Camera Angle"=w1077) -> (w1079:T2)
                  }
                  frame "GRT_ANG" {
                    n644 = Bundle By Name(cluster=w1082, "Grating Angle"=w1080) -> (w1081:T2)
                  }
                  frame "MOUNT_AZ" {
                    n645 = Bundle By Name(cluster=w1084, "Azimuth"=w1083) -> (w1085:T2)
                  }
                }
              }
              frame True {
              }
            }
          }
        }
        n646 = local write "Raw Data"(w1016) -> ()
      }
      frame "GET_IMAGE_STATS" {
        n647 = Array Size(array=w1091) -> (size(s)=w1090:i32[])
        n648 = Multiply Array Elements(1:w1090) -> (0:w1089:i32)
        n649 = Array Max & Min(array=w1091) -> (max value=→"Maximum Pix Value":i16, min value=→"Minimum Pix Value":i16)  [unwired: 2 out]
        n650 = Reshape Array(w1091, w1089) -> (w1088:i16[])
        n651 = To Double Precision Float(number=w1088) -> (double precision float=w1087:dbl[])
        n652 = Add Array Elements(numeric array=w1087) -> (sum=w1095:dbl)
        n653 = Divide(x=w1095, y=w1089) -> (x/y=→"Avg Pix Value":dbl)
      }
    }
    n654 = Equal?(x=w18, y="SHUTDOWN") -> (x = y?=w19:bool)
  }
  n655 = property on="Zoom Window" class="IntGraph (strict)" props=["X Scale", "Bounds:Area Width"]() -> ()  [unwired: 2 in, 3 out]
